vi "GCFS.vi"() -> ()   [LabVIEW 2024]
uses:
  Micro/DataCluster_GCFS.ctl
  <vilib>/userDefined/High Color/IMAQdx.ctl
  <vilib>/vision/Image Controls.llb/IMAQ Image.ctl
  <vilib>/DAQmx/read.llb/DAQmx Read (Analog DBL 1Chan 1Samp).vi
  a928a3f2-b033-44d4-bb12-0a68a29b5955.vi
  af9ea1de-6e94-45bd-9990-e3be68a33346.vi
  <vilib>/addons/_JKI Toolkits/State Machine/_JKI_lib_State_Machine.llb/Select State(s)_err__jki_lib_state_machine.vi
  acfa19c5-c678-4b0a-b648-770311154047.vi
  <extravilib>/ChannelInstances/Tag-t'DataCluster_GCFS.ctl'/Read With Abort.vi
  <extravilib>/ChannelInstances/Tag-t'DataCluster_GCFS.ctl'/Write With Abort.vi
  <extravilib>/ChannelInstances/Tag-t'DataCluster_GCFS.ctl'/Instantiate.vi
  <extravilib>/ChannelInstances/Tag-t'DataCluster_GCFS.ctl'/EndpointRead.vi
  <vilib>/DAQmx/miscellaneous.llb/DAQmx Fill In Error Info.vi
  <vilib>/addons/control/pid/pid.llb/PID (DBL).vi
  <vilib>/addons/_JKI Toolkits/State Machine/_JKI_lib_State_Machine.llb/Periodic Trigger__ogtk__JKI-SM__jki_lib_state_machine.vi
  <vilib>/Utility/file.llb/Write Delimited Spreadsheet (DBL).vi
  <vilib>/DAQmx/create/channels.llb/DAQmx Create Channel (AI-Temperature-RTD).vi
  <extravilib>/ChannelInstances/Tag-t'DataCluster_GCFS.ctl'/Endpoint.vi
  <vilib>/vision/driver/NI_Vision_Acquisition_Software.lvlib
  <extravilib>/ChannelInstances/Tag-t'DataCluster_GCFS.ctl'.lvlib
  <vilib>/addons/control/pid/NI_PID_pid.lvlib
panel:
  out "valid?":bool
  out "Waveform Chart":dbl(graph)
  in  "Load PID":bool
  in  "Tab Control":enum32{"Heating PID", "Cooling PID"}(tab)
  in  "proportional H":dbl=2.5
  in  "integral H":dbl=1.5
  in  "derivative H":dbl=0.8
  in  "proportional C":dbl=2.6
  in  "integral C":dbl=0.08
  in  "derivative C":dbl=0.1
  in  "OFF":bool
  in  "Cool":bool
  in  "Heat":bool
  in  "Cool A.":bool
  out "error out":errorcluster
  out "cDAQ Connection":bool
  out "Ready":bool
  in  "TempGrad":dbl=1.0
  in  "Get Temp":bool
  out "Temperature":dbl
  out "Data run":i32
  out "Droplet Lables":T1(plugin-control)
  in  "Grap Position Image":bool
  in  "Active":bool
  in  "Get Image":bool
  out "CAM Connection":bool
  out "UNO Connection":bool
  out "PSU Connection":bool
  out "Save loop":i32
  out "Data Loop":i32
  in  "Freezing value":sgl=250.0
  out "Frezz Image":T1(plugin-control)
  out "Droplet binary":T1(plugin-control)
  out "Grap Image":T1(plugin-control)
  in  "Sample name":string
  out "Statusstring":string
  out "Particle Measurements":dbl[][](array[numeric]) format="%.2f"
  out "Number of Particles":i32
  in  "Exit":bool
  # "Manual Controls"
  # "Temp"
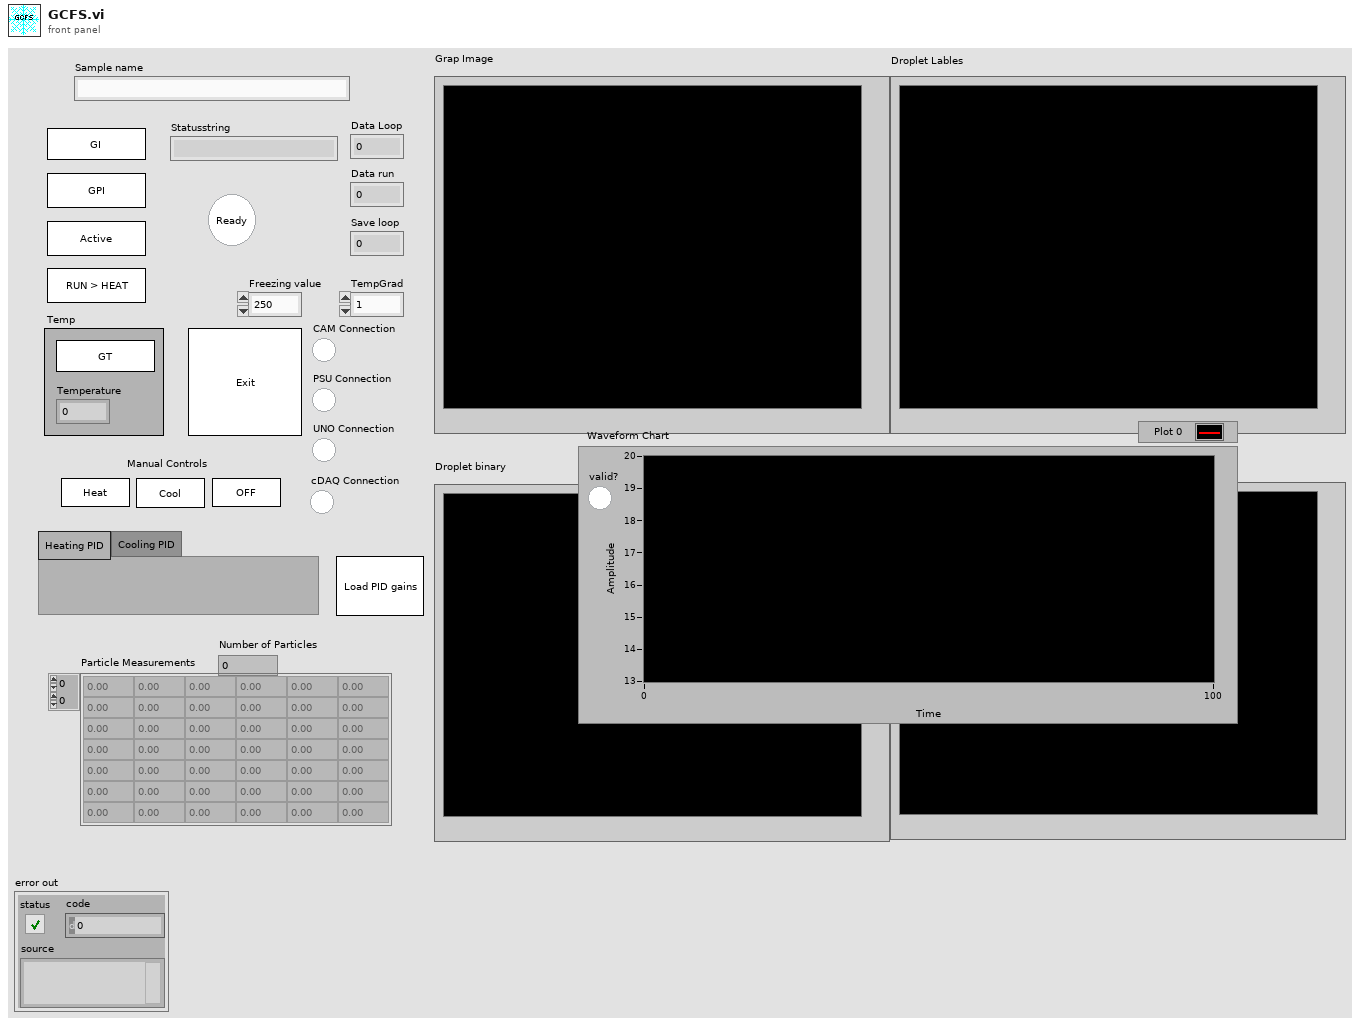
[diagram p1: front panel]
types:
  T1 = typedef "IMAQ Image.ctl" = refnum<image>
  T2 = typedef "DataCluster_GCFS.ctl" = cluster{"Core":cluster{"Current VI Reference":refnum<vi>, "Close Panel on Exit?":bool}, "Camera Cluster":cluster{"Session":T3, "Image":T1, "Position Image":T1, "PixelVal Image":T1, "Position Image Binary":T1, "Lable Image":T1, "Merged Image":T1, "Connection":bool}, "Data In Cluster":cluster{"Images":cluster{"Position Image path":path, "Sample folder path":path, "Label Image path":path}, "Sample Name":string, "Sample Rate":i32, "Gradient Buffer":i32, "Data Acquisition.Setup.TempGrad":dbl, "Control.HeatingPID gains":cluster{"proportional gain (Kc)":dbl, "integral time (Ti, min)":dbl, "derivative time (Td, min)":dbl}, "Freezing value":sgl, "Sample Rate 2":i32, "Control.CoolingPID gains":cluster{"proportional gain (Kc)":dbl, "integral time (Ti, min)":dbl, "derivative time (Td, min)":dbl}}, "Active":bool, "Ready":bool, "Exit":bool, "Arduino":cluster{"Connection":bool, "Port":refnum<visa-resource-name>, "State":string}, "Program_Start":string, "Data Out Cluster":cluster{"Particle Measurements":dbl[][], "Number of droplets":i32, "PosImg_Timestamp":string, "Que":refnum<queue>, "Lable coordinates":cluster{"X-Coordinate":i32, "Y-Coordinate":i32}[]}, "PSU":cluster{"Connection":bool, "Port":refnum<visa-resource-name>, "State":string}, "Load Rerun":bool, "Rerun":bool, "cDAQ":cluster{"Connection":bool, "ID":string, "Task":refnum<k21>}, "Temp":cluster{"Manual Temp":bool, "Target":dbl}, "Cool A.":bool}
  T3 = typedef "IMAQdx.ctl" = refnum<k21>
  T4 = enum32{"Invalid", "Standard", "Closed", "Hidden", "Minimized", "Maximized"}
  T5 = enum32{"invalid app kind", "Development System", "Run Time System", "Student Edition", "Embedded LabVIEW", "Evaluation", "Custom"}
  T6 = cluster{"Image To Save":T1, "Snap timestamp":string, "Pixel values":string[][], "Freezing points":string[][], "FreezingData":bool, "Image Pixels (U16)":u16[][]}
  T7 = cluster{"Current VI Reference":refnum<vi>, "Close Panel on Exit?":bool}
  T8 = cluster{"proportional gain (Kc)":dbl, "integral time (Ti, min)":dbl, "derivative time (Td, min)":dbl}
  T9 = typedef "Image Type" = u32
  T10 = cluster{"Type":u32, "Version":u32, "Flags":u32, "SerialNumberHigh":u32, "SerialNumberLow":u32, "BusType":u32, "InterfaceName":string, "VendorName":string, "ModelName":string, "CameraFileName":string, "CameraAttributeURL":string}[]
  T11 = typedef "Tag-t'DataCluster_GCFS.ctl'.lvlib/))Channel.ctl" = refnum<queue>
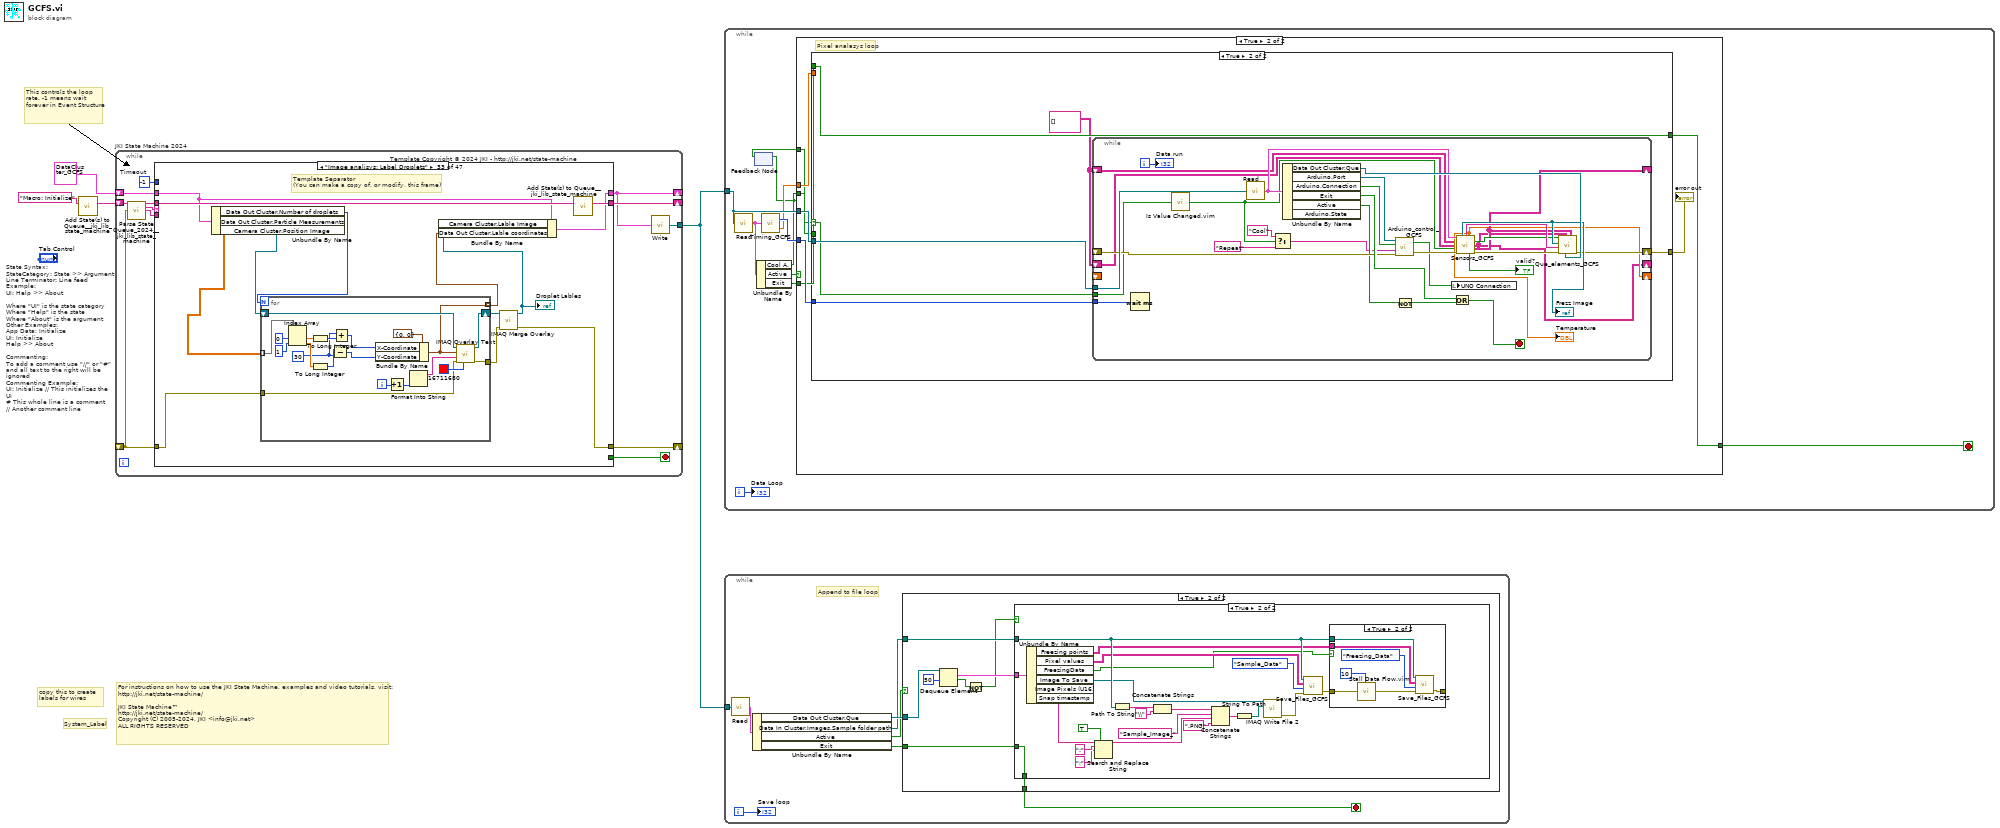
[diagram p0: block diagram]
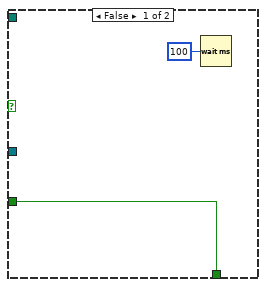
[diagram p2: hidden frame]
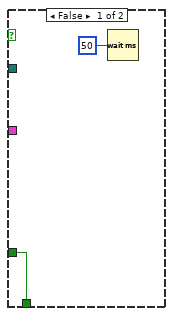
[diagram p3: hidden frame]
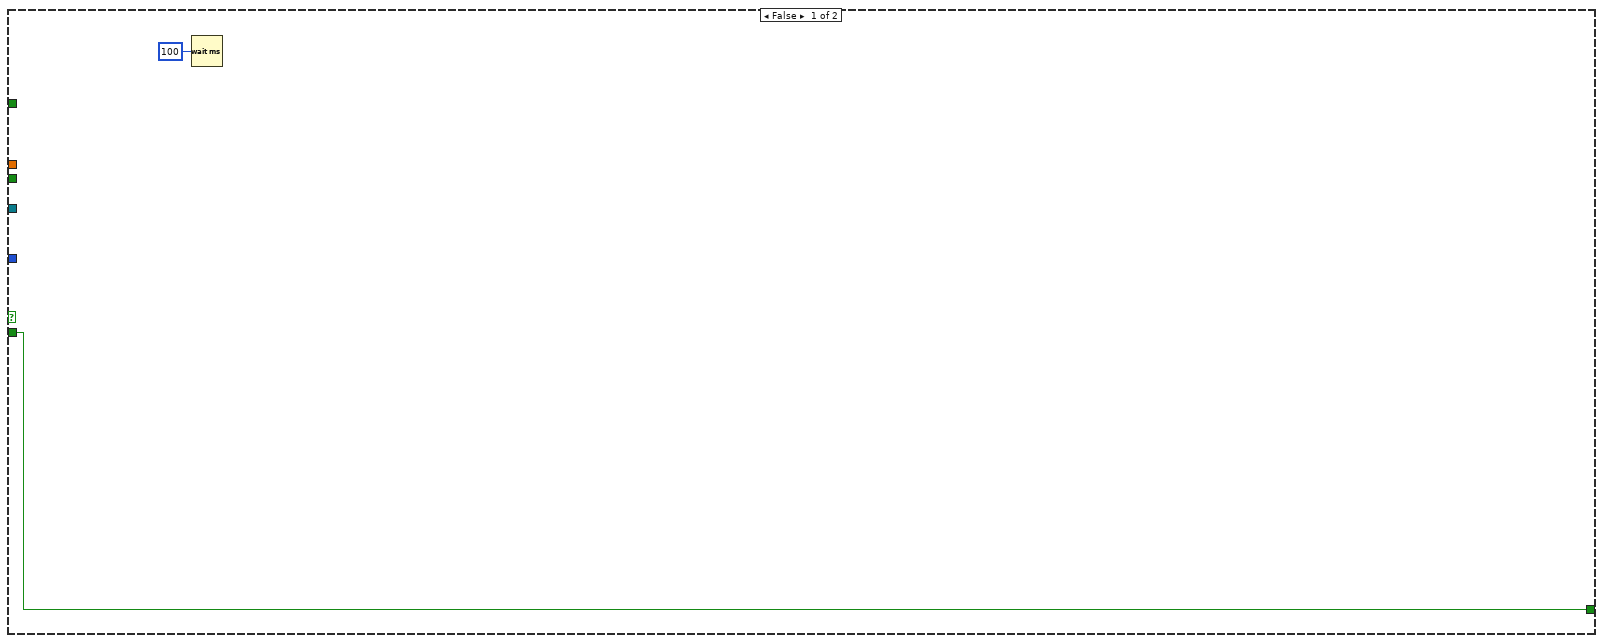
[diagram p5: hidden frame]
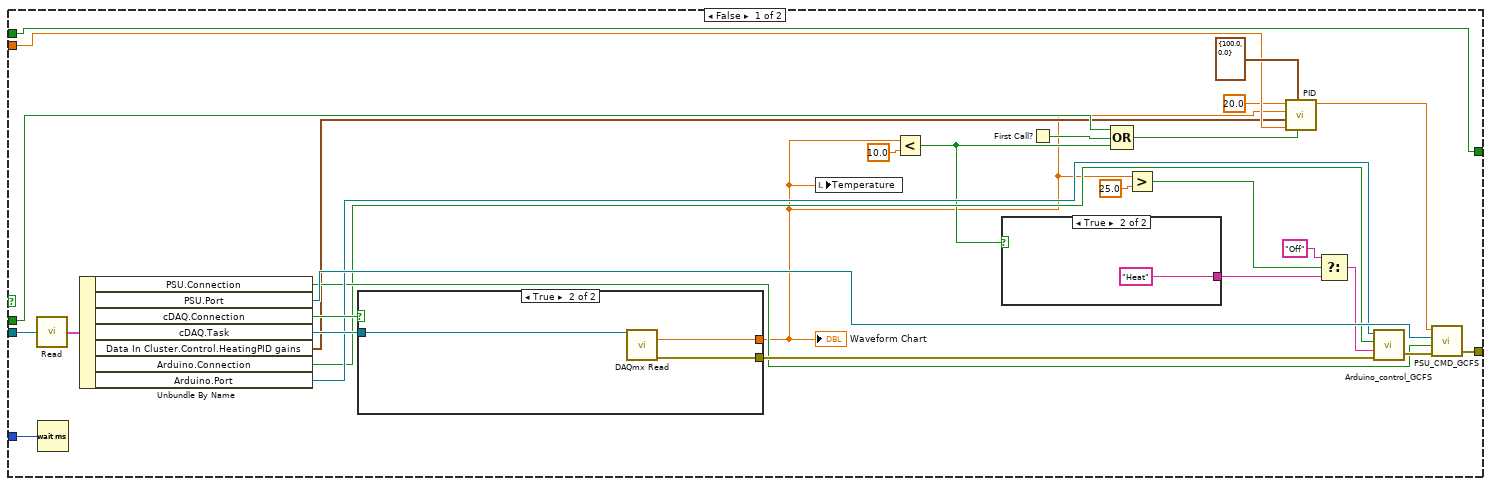
[diagram p6: hidden frame]
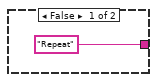
[diagram p7: hidden frame]
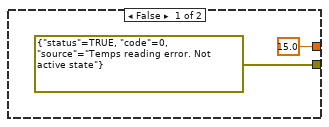
[diagram p8: hidden frame]
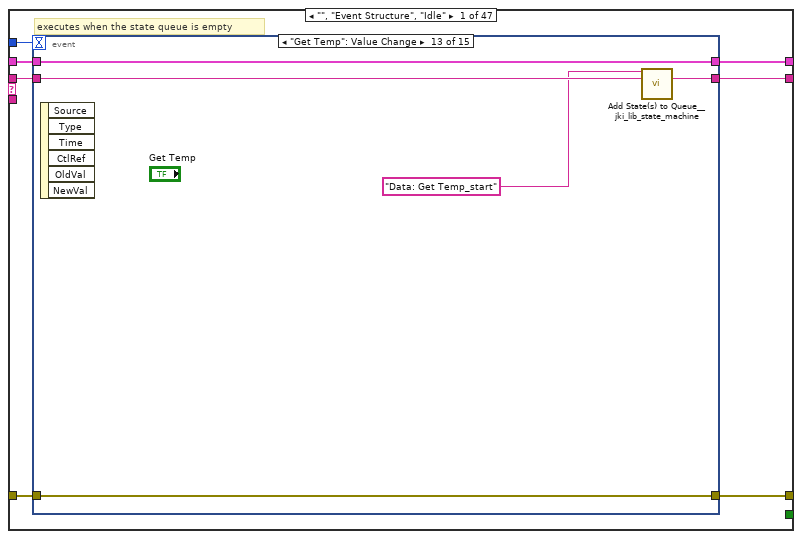
[diagram p9: hidden frame]
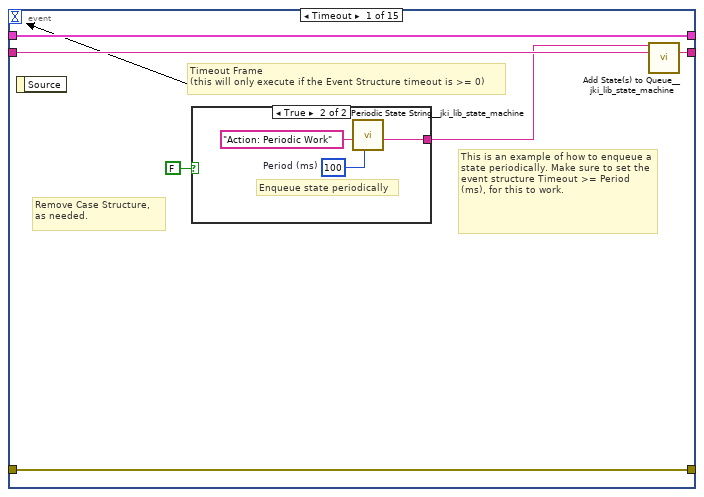
[diagram p10: hidden frame]
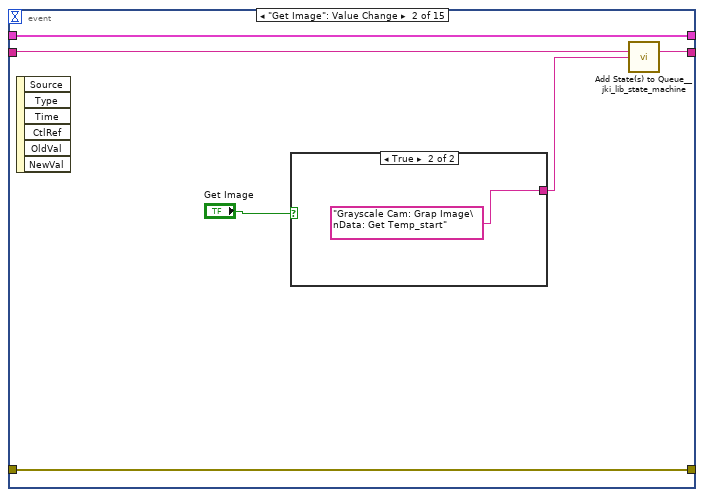
[diagram p12: hidden frame]
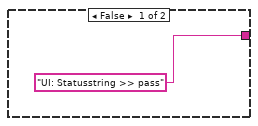
[diagram p13: hidden frame]
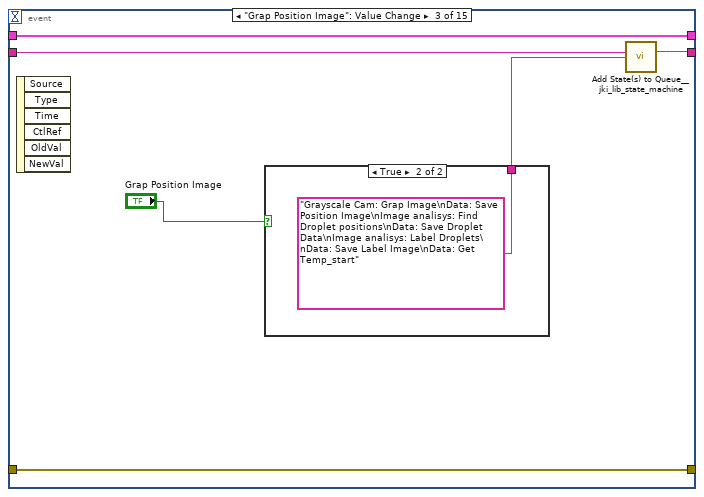
[diagram p14: hidden frame]
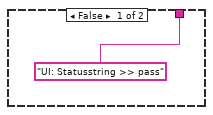
[diagram p15: hidden frame]
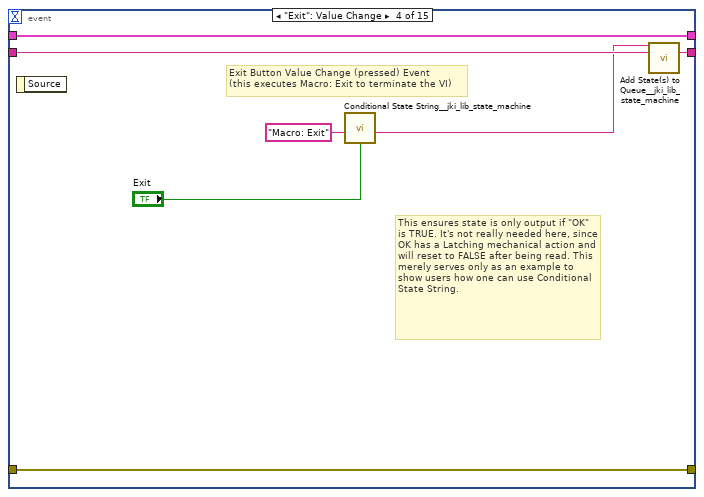
[diagram p16: hidden frame]
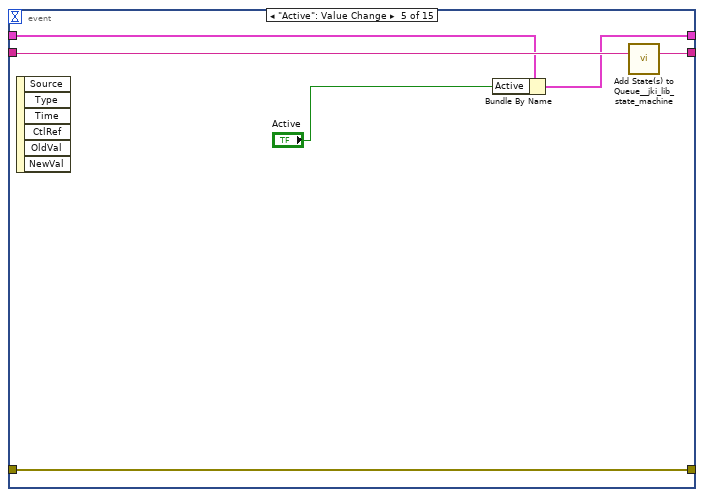
[diagram p17: hidden frame]
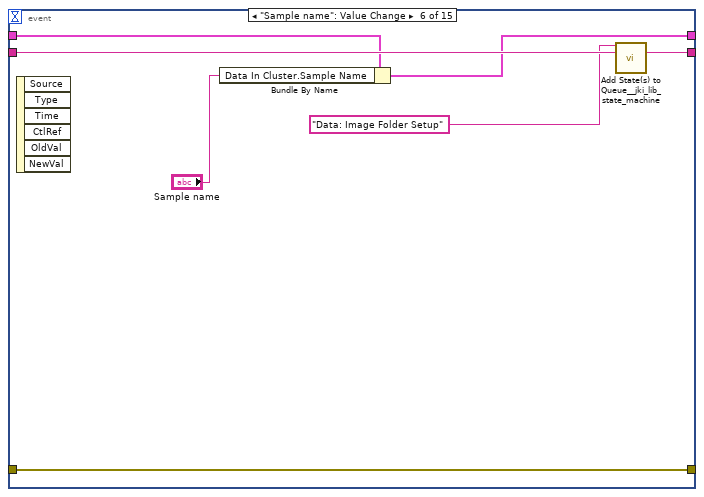
[diagram p18: hidden frame]
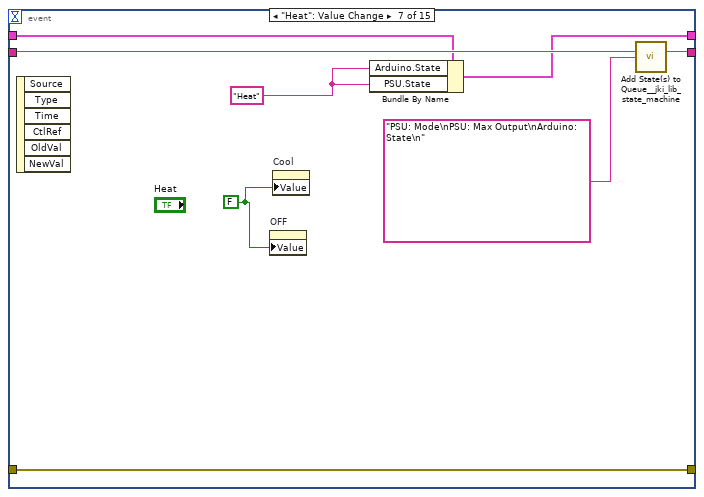
[diagram p19: hidden frame]
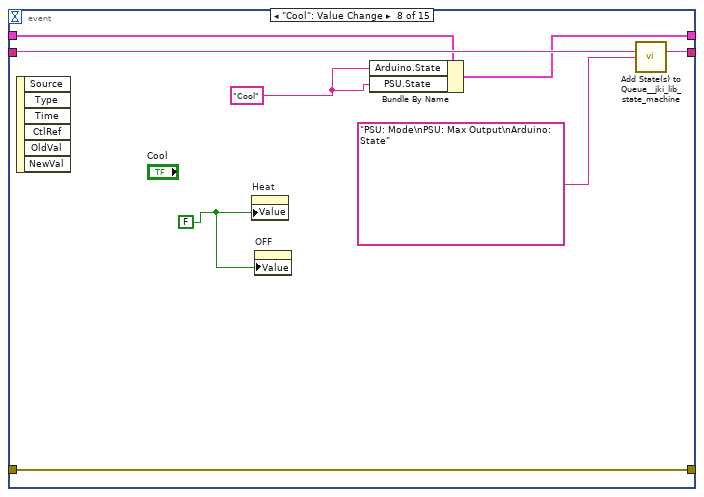
[diagram p20: hidden frame]
diagram:
  # "For instructions on how to use the JKI State Machine, examples and video tutorials, visit:\nhttp://jki.net/state-machine/\n\nJKI State Machine™\nhttp://jki.net/state-machine/\nCopyright (C) 2005-2024, JKI <info@jki.net>\nALL RIGHTS RESERVED"
  # "State Syntax:\nStateCategory: State >> Argument\nLine Terminator: Line feed\nExample:\nUI: Help >> About\n\nWhere \"UI\" is the state category\nWhere \"Help\" is the state\nWhere \"About\" is the argument\nOther Examples:\nApp Data: Initialize\nUI: Initialize\nHelp >> About\n\nCommenting:\nTo add a comment use \"//\" or \"#\" and all text to the right will be ignored\nCommenting Example:\nUI: Initialize // This initializes the UI\n# This whole line is a comment\n// Another comment line"
  # "copy this to create labels for wires"
  # "This controls the loop rate. -1 means wait forever in Event Structure"
  # "System_Label"
  n1 = call <vilib>:"Add State(s) to Queue__jki_lib_state_machine.vi"("State(s) in (\"\")"="Macro: Initialize") -> ("States Out"=w4:string)  [unwired: 14 in]
  n2 = while "JKI State Machine 2024" {
    shift-right: [w5] -> _
    shift-left: T2 {"Core"={"Current VI Reference"=refnum, "Close Panel on Exit?"=FALSE}, "Camera Cluster"={"Session"="", "Image"=refnum, "Position Image"=refnum, "PixelVal Image"=refnum, "Position Image Binary"=refnum, "Lable Image"=refnum, "Merged Image"=refnum, "Connection"=FALSE}, "Data In Cluster"={"Images"={"Position Image path"=path "", "Sample folder path"=path "", "Label Image path"=path ""}, "Sample Name"="", "Sample Rate"=20, "Gradient Buffer"=2, "Data Acquisition.Setup.TempGrad"=1.0, "Control.HeatingPID gains"={"proportional gain (Kc)"=2.5, "integral time (Ti, min)"=1.5, "derivative time (Td, min)"=0.8}, "Freezing value"=250.0, "Sample Rate 2"=20, "Control.CoolingPID gains"={"proportional gain (Kc)"=2.6, "integral time (Ti, min)"=0.08, "derivative time (Td, min)"=0.1}}, "Active"=FALSE, "Ready"=FALSE, "Exit"=FALSE, "Arduino"={"Connection"=FALSE, "Port"="", "State"=""}, "Program_Start"="", "Data Out Cluster"={"Particle Measurements"=[], "Number of droplets"=0, "PosImg_Timestamp"="", "Que"=refnum, "Lable coordinates"=[]}, "PSU"={"Connection"=FALSE, "Port"="", "State"=""}, "Load Rerun"=FALSE, "Rerun"=FALSE, "cDAQ"={"Connection"=FALSE, "ID"="", "Task"=""}, "Temp"={"Manual Temp"=FALSE, "Target"=0.0}, "Cool A."=FALSE} -> [w9]
    shift-right: [w12] -> _
    shift-left: _ -> [w7]
    shift-right: [w11] -> _
    shift-left: w4 -> [w13]
    tunnel: [w6] -> w1
    stop <- w10 stop-if-true
    w8 = -1  # Timeout
    # "Template Copyright © 2024 JKI - http://jki.net/state-machine"
    n3 = call <vilib>:"Parse State Queue_2024__jki_lib_state_machine.vi"("State Queue"=w13, "Error In (no error)"=w7) -> ("Remaining States"=w15:string, "Current State"=w16:string, "Arguments"=w14:string)  [unwired: 11 in]
    n4 = case shown="\"Image analisys: Label Droplets\"" w16 {
      selector: w16 -> [_ _ w131 _ _ _ _ _ _ _ _ _ _ _ _ _ _ _ _ _ _ _ _ _ _ _ _ _ _ _ _ _ _ _ _ _ _ _ _ _ _ _ _ _ _ _ _]
      tunnel: w15 -> [w23 w130 w135 w154 w164 w175 w179 w184 w195 w199 w213 w227 w232 w250 w270 w292 w308 w325 w329 w350 w354 w360 w371 w441 w446 w450 w465 w490 w515 w523 w535 w549 w562 w586 w594 w604 w612 w624 w632 w647 w656 w665 w674 w686 w696 w734 w742]
      tunnel: w14 -> [_ _ _ _ w159 _ _ _ _ _ _ _ _ _ _ _ _ _ _ _ _ w355 w365 w437 _ _ _ _ _ _ _ _ _ _ _ _ _ _ _ _ _ _ _ _ _ _ _]
      tunnel: w9 -> [w21 w127 w133 w147 w161 w171 w176 w181 w193 w196 w209 w224 w230 w245 w257 w282 w299 w323 w326 w348 w352 w358 w367 w438 w443 w447 w456 w481 w509 w518 w532 w545 w559 w583 w590 w600 w608 w621 w630 w643 w654 w663 w671 w683 w689 w719 w739]
      tunnel: [w20 w128 w137 w151 errorcluster {"status"=FALSE, "code"=0, "source"=""} ("error out") w173 w177 w182 w191 w197 w211 w225 w228 w246 w259 w283 w300 w309 w327 w342 w351 w356 w368 w439 w444 w448 w453 w483 w495 w520 w533 w546 w555 w584 w591 w596 w606 w622 w627 w641 w650 w659 w672 w684 w694 w716 w735] -> w12
      tunnel: w7 -> [w17 w128 w136 w151 w160 w173 w177 w182 w191 w197 w211 w225 w229 w247 w261 w284 w294 w310 w327 w344 w351 w357 w369 w439 w444 w448 w457 w485 w502 w519 w533 w537 w557 w584 w592 w597 w607 w622 w628 w642 w651 w660 w667 w684 w694 w717 w736]
      tunnel: [w22 w129 w134 w153 w163 w174 w178 w183 w194 w198 w212 w226 w231 w249 w269 w291 w307 w324 w328 w349 w353 w359 w370 w440 w445 w449 w464 w489 w514 w522 w534 w548 w561 w585 w593 w603 w611 w623 w631 w646 w655 w664 w673 w685 w695 w733 w741] -> w11
      tunnel: [_ _ _ _ _ TRUE _ _ _ _ _ _ _ _ _ _ _ _ _ _ _ _ _ _ _ _ _ _ _ _ _ _ _ _ _ _ _ _ _ _ _ _ _ _ _ _ _] -> w10
      tunnel: [w19 w127 w133 w152 w161 w170 w176 w181 w193 w196 w208 w223 w230 w245 w256 w281 w298 w323 w326 w348 w352 w358 w367 w438 w443 w447 w455 w482 w513 w521 w532 w544 w558 w583 w589 w599 w605 w621 w629 w643 w654 w663 w671 w683 w688 w718 w740] -> w5
      tunnel: w8 -> [w18 _ _ _ _ _ _ _ _ _ _ _ _ _ _ _ _ _ _ _ _ _ _ _ _ _ _ _ _ _ _ _ _ _ _ _ _ _ _ _ _ _ _ _ _ _ _]
      frame "", "Event Structure", "Idle" {
        # "executes when the state queue is empty"
        n5 = event shown="[12] \"Get Temp\": Value Change" {
          selector: _ -> [_ _ _ _ _ _ _ _ _ _ _ _ _ _ _]
          dyn-events: _ -> [_ _ _ _ _ _ _ _ _ _ _ _ _ _ _]
          timeout: w18 -> [_ _ _ _ _ _ _ _ _ _ _ _ _ _ _]
          tunnel: w23 -> [w29 w35 w44 w55 w60 w67 w75 w83 w91 w97 w100 w109 w112 w119 w125]
          tunnel: [w28 w36 w45 w54 w61 w68 w76 w84 w92 w98 w101 w108 w111 w120 w126] -> w22
          tunnel: w21 -> [w26 w37 w46 w52 w59 w65 w73 w81 w89 w95 w103 w106 w114 w116 w123]
          tunnel: [w27 w38 w41 w53 w56 w62 w74 w82 w90 w96 w102 w107 w113 w118 w121] -> w20
          tunnel: w17 -> [w27 w38 w41 w53 w56 w62 w74 w82 w90 w96 w102 w107 w113 w118 w121]
          tunnel: [w26 w37 w46 w52 w58 w64 w72 w80 w88 w94 w103 w106 w114 w117 w124] -> w19
          event Timeout {
            # "Remove Case Structure, as needed."
            # "This is an example of how to enqueue a state periodically. Make sure to set the event structure Timeout >= Period (ms), for this to work."
            # "Timeout Frame\n(this will only execute if the Event Structure timeout is >= 0)"
            n6 = event-data() -> ()  [unwired: 1 in, 1 out]
            n7 = case shown="True" FALSE {
              tunnel: [_ w32] -> w25
              frame False {
              }
              frame True {
                w30 = u32 100  # Period (ms)
                # "Enqueue state periodically"
                n8 = call <vilib>:"Periodic State String__jki_lib_state_machine.vi"("Period (ms)"=w30, "State"="Action: Periodic Work") -> ("State Out"=w32:string)  [unwired: 9 in]
              }
            }
            n9 = call <vilib>:"Add State(s) to Queue__jki_lib_state_machine.vi"("State(s) in Front (\"\")"=w25, "State(s) in (\"\")"=w29) -> ("States Out"=w28:string)  [unwired: 13 in]
          }
          event "Get Image": Value Change {
            n10 = event-data() -> ()  [unwired: 1 in, 6 out]
            n11 = case shown="True" "Get Image" {
              tunnel: ["UI: Statusstring >> pass" "Grayscale Cam: Grap Image\nData: Get Temp_start"] -> w34
              frame False {
              }
              frame True {
              }
            }
            n12 = call <vilib>:"Add State(s) to Queue__jki_lib_state_machine.vi"("State(s) in (\"\")"=w35, "State(s) at Back (\"\")"=w34) -> ("States Out"=w36:string)  [unwired: 13 in]
          }
          event "Grap Position Image": Value Change {
            n13 = event-data() -> ()  [unwired: 1 in, 6 out]
            n14 = case shown="True" "Grap Position Image" {
              tunnel: ["UI: Statusstring >> pass" "Grayscale Cam: Grap Image\nData: Save Position Image\nImage analisys: Find Droplet positions\nData: Save Droplet Data\nImage analisys: Label Droplets\nData: Save Label Image\nData: Get Temp_start"] -> w42
              frame False {
              }
              frame True {
              }
            }
            n15 = call <vilib>:"Add State(s) to Queue__jki_lib_state_machine.vi"("State(s) in (\"\")"=w44, "State(s) at Back (\"\")"=w42) -> ("States Out"=w45:string)  [unwired: 13 in]
          }
          event "Exit": Value Change {
            # "This ensures state is only output if \"OK\" is TRUE. It's not really needed here, since OK has a Latching mechanical action and will reset to FALSE after being read. This merely serves only as an example to show users how one can use Conditional State String."
            # "Exit Button Value Change (pressed) Event\n(this executes Macro: Exit to terminate the VI)"
            n16 = event-data() -> ()  [unwired: 1 in, 1 out]
            n17 = call <vilib>:"Conditional State String__jki_lib_state_machine.vi"("Do State(s)?"="Exit", "State"="Macro: Exit") -> ("State Out"=w49:string)  [unwired: 7 in]
            n18 = call <vilib>:"Add State(s) to Queue__jki_lib_state_machine.vi"("State(s) in Front (\"\")"=w49, "State(s) in (\"\")"=w55) -> ("States Out"=w54:string)  [unwired: 13 in]
          }
          event "Active": Value Change {
            n19 = event-data() -> ()  [unwired: 1 in, 6 out]
            n20 = Bundle By Name(cluster=w59, "Active"="Active") -> (w58:T2)
            n21 = call <vilib>:"Add State(s) to Queue__jki_lib_state_machine.vi"("State(s) in (\"\")"=w60) -> ("States Out"=w61:string)  [unwired: 14 in]
          }
          event "Sample name": Value Change {
            n22 = event-data() -> ()  [unwired: 1 in, 6 out]
            n23 = Bundle By Name(cluster=w65, "Data In Cluster.Sample Name"="Sample name") -> (w64:T2)
            n24 = call <vilib>:"Add State(s) to Queue__jki_lib_state_machine.vi"("State(s) in Front (\"\")"="Data: Image Folder Setup", "State(s) in (\"\")"=w67) -> ("States Out"=w68:string)  [unwired: 13 in]
          }
          event "Heat": Value Change {
            w71 = FALSE
            w69 = "Heat" ("Arduino.State")
            n25 = event-data() -> ()  [unwired: 1 in, 6 out]
            n26 = property on="OFF" class="Bool (strict)"("Value"=w71) -> ()  [unwired: 2 in, 2 out]
            n27 = property on="Cool" class="Bool (strict)"("Value"=w71) -> ()  [unwired: 2 in, 2 out]
            n28 = Bundle By Name(cluster=w73, "Arduino.State"=w69, "PSU.State"=w69) -> (w72:T2)
            n29 = call <vilib>:"Add State(s) to Queue__jki_lib_state_machine.vi"("State(s) in (\"\")"=w75, "State(s) at Back (\"\")"="PSU: Mode\nPSU: Max Output\nArduino: State\n") -> ("States Out"=w76:string)  [unwired: 13 in]
          }
          event "Cool": Value Change {
            w79 = FALSE
            w77 = "Cool" ("Arduino.State")
            n30 = event-data() -> ()  [unwired: 1 in, 6 out]
            n31 = property on="Heat" class="Bool (strict)"("Value"=w79) -> ()  [unwired: 2 in, 2 out]
            n32 = property on="OFF" class="Bool (strict)"("Value"=w79) -> ()  [unwired: 2 in, 2 out]
            n33 = Bundle By Name(cluster=w81, "Arduino.State"=w77, "PSU.State"=w77) -> (w80:T2)
            n34 = call <vilib>:"Add State(s) to Queue__jki_lib_state_machine.vi"("State(s) in (\"\")"=w83, "State(s) at Back (\"\")"="PSU: Mode\nPSU: Max Output\nArduino: State") -> ("States Out"=w84:string)  [unwired: 13 in]
          }
          event "OFF": Value Change {
            w87 = FALSE
            w85 = "OFF" ("Arduino.State")
            n35 = event-data() -> ()  [unwired: 1 in, 6 out]
            n36 = property on="Cool" class="Bool (strict)"("Value"=w87) -> ()  [unwired: 2 in, 2 out]
            n37 = property on="Heat" class="Bool (strict)"("Value"=w87) -> ()  [unwired: 2 in, 2 out]
            n38 = Bundle By Name(cluster=w89, "Arduino.State"=w85, "PSU.State"=w85) -> (w88:T2)
            n39 = call <vilib>:"Add State(s) to Queue__jki_lib_state_machine.vi"("State(s) in (\"\")"=w91, "State(s) at Back (\"\")"="PSU: Min Output\nPSU: Mode\nArduino: State") -> ("States Out"=w92:string)  [unwired: 13 in]
          }
          event "Cool A.": Value Change {
            n40 = event-data() -> ()  [unwired: 1 in, 6 out]
            n41 = Bundle By Name(cluster=w95, "Cool A."="Cool A.") -> (w94:T2)
            n42 = call <vilib>:"Add State(s) to Queue__jki_lib_state_machine.vi"("State(s) in (\"\")"=w97) -> ("States Out"=w98:string)  [unwired: 14 in]
          }
          event "Load PID": Value Change {
            n43 = event-data() -> ()  [unwired: 1 in, 6 out]
            n44 = call <vilib>:"Add State(s) to Queue__jki_lib_state_machine.vi"("State(s) in Front (\"\")"="Data: PID gains" ("State(s) in Front (\"\")"), "State(s) in (\"\")"=w100) -> ("States Out"=w101:string)  [unwired: 13 in]
          }
          event Panel Close? {
            # "Discard the event because we'll close the front panel ourselves in Macro: Exit"
            # "Close Panel button (pressed) Event\n(this executes Macro: Exit to terminate the VI)"
            n45 = event-data() -> ()  [unwired: 1 in, 1 out]
            n46 = event-data("Discard?"=TRUE) -> ()  [unwired: 1 in, 1 out]
            n47 = call <vilib>:"Add State(s) to Queue__jki_lib_state_machine.vi"("State(s) in Front (\"\")"="Macro: Exit", "State(s) in (\"\")"=w109) -> ("States Out"=w108:string)  [unwired: 13 in]
          }
          event "Get Temp": Value Change {
            n48 = event-data() -> ()  [unwired: 1 in, 6 out]
            n49 = call <vilib>:"Add State(s) to Queue__jki_lib_state_machine.vi"("State(s) in Front (\"\")"="Data: Get Temp_start" ("State(s) in Front (\"\")"), "State(s) in (\"\")"=w112) -> ("States Out"=w111:string)  [unwired: 13 in]
          }
          event "TempGrad": Value Change {
            n50 = event-data() -> ()  [unwired: 1 in, 6 out]
            n51 = Bundle By Name(cluster=w116, "Data In Cluster.Data Acquisition.Setup.TempGrad"="TempGrad") -> (w117:T2)
            n52 = call <vilib>:"Add State(s) to Queue__jki_lib_state_machine.vi"("State(s) in (\"\")"=w119) -> ("States Out"=w120:string)  [unwired: 14 in]
          }
          event "Freezing value": Value Change {
            n53 = event-data() -> ()  [unwired: 1 in, 6 out]
            n54 = Bundle By Name(cluster=w123, "Data In Cluster.Freezing value"="Freezing value") -> (w124:T2)
            n55 = call <vilib>:"Add State(s) to Queue__jki_lib_state_machine.vi"("State(s) in (\"\")"=w125) -> ("States Out"=w126:string)  [unwired: 14 in]
          }
        }
      }
      frame "---------- Core ----------" {
        # "Do not put any code in this frame.\n(it is a separator no-op)"
        n56 = call <vilib>:"Add State(s) to Queue__jki_lib_state_machine.vi"("State(s) in (\"\")"=w130) -> ("States Out"=w129:string)  [unwired: 14 in]
      }
      frame Default {
        w140 = 42 items=["No error", "Argument error", "Memory is full", "Out of zone", "End of file", "File already open", "Generic file I/O error", "File not found", "File permission error", "Disk is full", "Duplicate path", "Too many files open", "System feature not enabled", "Resource file not found", "Cannot add resource", "Resource not found", "Image not found", "Image memory error", "Pen does not exist", "Config type invalid", "Config token not found", "Config parse error", "Config memory error", "Bad external code format", "Bad external code offset", "External code not present", "Null window", "Destroy window error", "Null menu", "Print aborted", "Bad print record", "Print driver error", "Windows error during printing", "Memory error during printing", "Print dialog error", "Generic print error", "Invalid device refnum", "Device not found", "Device parameter error", "Device unit error", "Cannot open device", "Device call aborted", "Generic error", "Cancelled by user", "Object ID too low", "Object ID too high", "Object not in heap", "Unknown heap", "Unknown object (invalid DefProc)", "Unknown object (DefProc not in table)", "Message out of range", "Invalid (null) method", "Unknown message", "Manager call not supported", "Bad address", "Network operation in progress", "Network operation timed out", "Connection is busy", "Network attribute not supported", "Network error", "Address in use", "System out of memory", "Connection aborted", "Connection refused", "Not connected", "Already connected", "Connection closed", "Initialization error (interapplication manager)", "Bad occurrence", "Wait on unbound occurrence handler", "Occurrence queue overflow", "Datalog type conflict", "Unused", "Unrecognized type (interapplication manager)", "Memory corrupt", "Failed to make temporary DLL", "Old CIN version", "Drag socket not found", "Failed to load drop-object", "Failed to register OLE object", "Failed to release OLE object", "Format specifier type mismatch", "Unknown format specifier", "Too few format specifiers", "Too many format specifiers", "Scan failed", "Newer CIN version", "Error converting to variant", "Runtime menu error", "Password tampered", "Variant attribute not found", "Incompatible variant data type", "Event data is not available", "Event Store is not present", "Occurrence is not found", "Event Queue is not created", "Event info is not available", "Refnum passed is NULL", "Error retrieving Class GUID", "Error retrieving CoClass GUID", "Error retrieving TypeLib GUID.", "Bad built application magic bytes.", "Specific driver is different from the specific driver associated with the Logical Name.", "There is no session opened to the class driver.", "Max Error", "MAX - Error with config objects", "MAX - Error loading configuration", "MAX - Group not supported"]
        # "Current State"
        # "Do not delete, rename, or modify this frame.\n(this is used to capture unhandled states and typos)"
        # "Handle mistyped state name (developer tool)"
        n57 = Format Into String(format string="Software Exception: Unhandled State \"%s\"." ("message"), error in=w136, w131) -> (resulting string=w139:string, error out=w138:errorcluster)  [unwired: 1 in]
        n58 = call <vilib>:"Error Cluster From Error Code.vi"("show call chain? (False)"=TRUE, "error in (no error)"=w138, "error message (\"\")"=w139, "error code (0)"=w140) -> ("error out"=w137:errorcluster)  [unwired: 5 in]
        n59 = call <vilib>:"Add State(s) to Queue__jki_lib_state_machine.vi"("State(s) in (\"\")"=w135) -> ("States Out"=w134:string)  [unwired: 14 in]
      }
      frame "Initialize Core Data" {
        # "Do not delete, rename, or modify this frame.\n(this is used to determine panel behavior on exit)"
        # "originally closed?"
        # "exe?"
        # "If panel starts closed or is an EXE, then close it when we exit"
        n60 = property class="VI"() -> ("FP.State"=w144:T4)  [unwired: 2 in, 2 out]
        n61 = property class="App"() -> ("App.Kind"=w150:T5)  [unwired: 2 in, 2 out]
        n62 = control-ref of="Current VI Reference"() -> (w145:refnum<vi>)
        n63 = Equal?(x=w144, y=T4."Closed" ("Front Panel Window:State")) -> (x = y?=w142:bool)
        n64 = Equal?(x=w150, y=T5."Run Time System" ("Application:Kind")) -> (x = y?=w148:bool)
        n65 = Or(x=w142, y=w148) -> (x .or. y?=w146:bool)
        n66 = Bundle By Name(cluster=w147, "Core.Current VI Reference"=w145, "Core.Close Panel on Exit?"=w146) -> (w152:T2)
        n67 = call <vilib>:"Add State(s) to Queue__jki_lib_state_machine.vi"("State(s) in (\"\")"=w154) -> ("States Out"=w153:string)  [unwired: 14 in]
      }
      frame "Error Handler" {
        # "When running as sourcecode, this function will add previous state data to the error message to aid the developer in troubleshoot errors.\nIf run as an executable, no additional information is added to the error message."
        # "This state receives both Errors and Warnings which is how the Status of this wire can be FALSE"
        # "Unhandled Error -- Display it"
        # "Handle any errors or warnings here.\nYou can also output any states to clean-up after errors or warnings occur"
        # "Clear error or warning"
        n68 = disable-structure shown="Default" {
          disable-tunnel: w160 -> [w167 w168]
          disable-tunnel: w159 -> [w166 _]
          disable-tunnel: [w165 w168] -> w158
          frame condition #0 (active) {
            n69 = call <vilib>:"Append Error Details__jki_lib_state_machine.vi"("error in (no error)"=w167, "Previous State and Argument(s)"=w166) -> ("error out"=w165:errorcluster)  [unwired: 9 in]
          }
          frame condition #1 {
          }
        }
        n70 = call <vilib>:"General Error Handler.vi"("error in (no error)"=w158) -> ()  [unwired: 10 in, 5 out]
        n71 = call-poly <vilib>:"Select State(s)__jki_lib_state_machine.vi"("State(s) if True (\"\")"="/* Post Error States", "Select"=w158, "State(s) if False (\"\")"="/* Post Warning States") -> ("States Out"=w156:string)  [unwired: 12 in]
        n72 = call <vilib>:"Add State(s) to Queue__jki_lib_state_machine.vi"("State(s) in Front (\"\")"=w156, "State(s) in (\"\")"=w164) -> ("States Out"=w163:string)  [unwired: 13 in]
      }
      frame "Exit" {
        # "Do not put any code in this frame.\n(No errors that occur here will be handled.)"
        n73 = Bundle By Name(cluster=w171, "Exit"=TRUE) -> (w170:T2)
        n74 = call <vilib>:"Add State(s) to Queue__jki_lib_state_machine.vi"("State(s) in (\"\")"=w175) -> ("States Out"=w174:string)  [unwired: 14 in]
      }
      frame "---------- Macro ----------" {
        # "Do not put any code in this frame.\n(It is a separator no-op. You can make a copy of this frame to create a new Macro frame)"
        n75 = call <vilib>:"Add State(s) to Queue__jki_lib_state_machine.vi"("State(s) in (\"\")"=w179) -> ("States Out"=w178:string)  [unwired: 14 in]
      }
      frame "Macro: Initialize" {
        w180 = "UI: Initialize\nUI: Statusstring >> Initialysing\ncDAQ: Scan\ncDAQ: Initialize\nPSU: Initialize\nPSU: Mode\nArduino: Initialize\nGrayscale Cam: Initialize\nData: Initialize\nData: PID gains\nInitialize Core Data\nUI: Front Panel State >> Open\nData: Get Temp_start\nData: Image Folder Setup\nUI: Statusstring >> Initialysation done\nUI: Ready"  # UI: Initialize UI: Statusstring >> Initialysing cDAQ: Scan cDAQ: Initialize PSU: Initialize PSU: Mode Arduino: Initialize Grayscale Cam: Initialize Data: Initialize Data: PID gains Initialize Core Data UI: Front Panel State >> Open Data: Get Temp_start Data: Image Folder Setup UI: Statusstring >> Initialysation done UI: Ready
        # "Initialization Macro\n(This is called once, when the VI starts)"
        n76 = call <vilib>:"Add State(s) to Queue__jki_lib_state_machine.vi"("State(s) in Front (\"\")"=w180, "State(s) in (\"\")"=w184) -> ("States Out"=w183:string)  [unwired: 13 in]
      }
      frame "Macro: Exit" {
        w192 = "Data: Cleanup\nUI: StatusString >> Terminating cDAQ Connection (Thermistor)\ncDAQ: Terminate\nUI: StatusString >> Terminating Camera Connection\nGrayscale Cam: Terminate\nUI: StatusString >> Terminating Arduino Connection\nArduino: Terminate\nUI: StatusString >> Terminating Power Supply\nPSU: Terminate\nUI: StatusString >> See you soon\nUI: Uninitialize\nExit"  # Data: Cleanup UI: StatusString >> Terminating cDAQ Connection (Thermistor) cDAQ: Terminate UI: StatusString >> Terminating Camera Connection Grayscale Cam: Terminate UI: StatusString >> Terminating Arduino Connection Arduino: Terminate UI: StatusString >> Terminating Power Supply PSU: Terminate UI: StatusString >> See you soon UI: Uninitialize Exit
        # "Exit Macro\n(This is called once, when the VI exits)"
        n77 = Unbundle By Name(w193) -> ("Core.Close Panel on Exit?"=w189:bool)
        n78 = call <vilib>:"Conditional State String__jki_lib_state_machine.vi"("Do State(s)?"=w189, "State"="UI: Front Panel State >> Close") -> ("State Out"=w188:string)  [unwired: 7 in]
        n79 = call <vilib>:"Add State(s) to Queue__jki_lib_state_machine.vi"("State(s) in (\"\")"=w188, "State(s) at Back (\"\")"=w192) -> ("States Out"=w187:string)  [unwired: 13 in]
        n80 = call "Stall Data Flow.vim"("value in"=w187, "milliseconds to wait"=u32 50) -> ("value out"=w186:string)  [unwired: 1 out]
        n81 = call <vilib>:"Add State(s) to Queue__jki_lib_state_machine.vi"("State(s) in Front (\"\")"=w186, "State(s) in (\"\")"=w195) -> ("States Out"=w194:string)  [unwired: 13 in]
      }
      frame "---------- Data ----------" {
        # "Do not put any code in this frame.\n(It is a separator no-op. You can make a copy of this frame to create a new Data frame)"
        n82 = call <vilib>:"Add State(s) to Queue__jki_lib_state_machine.vi"("State(s) in (\"\")"=w199) -> ("States Out"=w198:string)  [unwired: 14 in]
      }
      frame "Data: Initialize" {
        w210 = T7 {"Current VI Reference"=refnum, "Close Panel on Exit?"=FALSE}  # Core
        # "do not delete - used by framework"
        # "Initialize the shift-register data, here.\n(data names are defined by what you wire into the bundle function)"
        n83 = local read "Sample name"() -> (w206:string)
        n84 = Equal?(x=w206, y="") -> (x = y?=w205:bool)
        n85 = call "Prompt User for Sample name"("Enable"=w205) -> ("Sample name"=w204:string)  [unwired: 16 in, 2 out]
        n86 = Select(t=w204, s=w205, f=w206) -> (s? t:f=w203:string)
        n87 = Obtain Queue(name (unnamed)="Save Queue", element data type=T6 {"Image To Save"=refnum, "Snap timestamp"="", "Pixel values"=[], "Freezing points"=[], "FreezingData"=FALSE, "Image Pixels (U16)"=[]}) -> (queue out=w200:refnum<queue>)  [unwired: 3 in, 2 out]
        n88 = Bundle By Name(cluster=w209, "Data Out Cluster.Que"=w200, "Core"=w210, "Data In Cluster.Sample Name"=w203) -> (w208:T2)
        n89 = local write "Sample name"(w203) -> ()
        n90 = call <vilib>:"Add State(s) to Queue__jki_lib_state_machine.vi"("State(s) in (\"\")"=w213) -> ("States Out"=w212:string)  [unwired: 14 in]
      }
      frame "Data: PID gains" {
        w222 = T8 {"proportional gain (Kc)"=0.0, "integral time (Ti, min)"=0.0, "derivative time (Td, min)"=0.0} ("Data In Cluster.Control.HeatingPID gains")
        # "Do not put any code in this frame.\n(It is a separator no-op. You can make a copy of this frame to create a new Data frame)"
        n91 = Bundle By Name(cluster=w222, "proportional gain (Kc)"="proportional H", "integral time (Ti, min)"="integral H", "derivative time (Td, min)"="derivative H") -> (w221:T8)
        n92 = Bundle By Name(cluster=w222, "proportional gain (Kc)"="proportional C", "integral time (Ti, min)"="integral C", "derivative time (Td, min)"="derivative C") -> (w220:T8)
        n93 = Bundle By Name(cluster=w224, "Data In Cluster.Control.HeatingPID gains"=w221, "Data In Cluster.Control.CoolingPID gains"=w220) -> (w223:T2)
        n94 = call <vilib>:"Add State(s) to Queue__jki_lib_state_machine.vi"("State(s) in (\"\")"=w227) -> ("States Out"=w226:string)  [unwired: 14 in]
      }
      frame "Data: Get Temp_start" {
        # "Do not put any code in this frame.\n(It is a separator no-op. You can make a copy of this frame to create a new Data frame)"
        n95 = disable-structure shown="Enabled" {
          disable-tunnel: w230 -> [_ w239]
          disable-tunnel: w229 -> [_ w236]
          disable-tunnel: [_ w235] -> w228
          frame Disabled {
            n96 = call "DAQ Assistant"("timeout (s)"=0.5) -> ("data"=w233:dynamicdata)  [unwired: 16 in, 2 out]
            n97 = local write "Temperature"(w233) -> ()
          }
          frame Enabled {
            n98 = Unbundle By Name(w239) -> ("cDAQ.Task"=w238:refnum<k21>, "cDAQ.Connection"=w237:bool)
            n99 = case shown="True" w237 {
              tunnel: w238 -> [_ w244]
              tunnel: w236 -> [w240 w243]
              tunnel: [w240 w242] -> w235
              frame False {
              }
              frame True {
                n100 = call-poly <vilib>:"DAQmx Read.vi"("task/channels in"=w244, "error in"=w243) -> ("data"=w241:dbl, "error out"=w242:errorcluster)  [unwired: 11 in, 1 out]
                n101 = local write "Temperature"(w241) -> ()
              }
            }
          }
        }
        n102 = call <vilib>:"Add State(s) to Queue__jki_lib_state_machine.vi"("State(s) in (\"\")"=w232) -> ("States Out"=w231:string)  [unwired: 14 in]
      }
      frame "Data: Cleanup" {
        # "Cleanup any data and references, here.\n(this is called automatically, by the Macro: Exit)"
        n103 = Unbundle By Name(w245) -> ("Core.Current VI Reference"=w248:refnum<vi>)
        n104 = Close Reference(reference=w248, error in (no error)=w247) -> (error out=w246:errorcluster)
        n105 = call <vilib>:"Add State(s) to Queue__jki_lib_state_machine.vi"("State(s) in (\"\")"=w250) -> ("States Out"=w249:string)  [unwired: 14 in]
      }
      frame "Data: Image Folder Setup" {
        w252 = "\\" ("string")
        # "Do not put any code in this frame.\n(It is a separator no-op. You can make a copy of this frame to create a new Data frame)"
        n106 = Unbundle By Name(w257) -> ("Data In Cluster.Sample Name"=w258:string)
        n107 = Format Date/Time String(time format string (%c)="%Y-%m-%d_%H;%M", UTC format=FALSE) -> (date/time string=w251:string)  [unwired: 1 in]
        n108 = call <vilib>:"Application Directory.vi"() -> ("Application Directory"=w267:path)
        n109 = Path To String(path=w267) -> (string=w266:string)
        n110 = Concatenate Strings(w266, w252, "Flat Surface Images" ("string"), w252, w258, w252, w251) -> (w264:string)
        n111 = String To Path(string=w264) -> (path=w265:path)
        n112 = call <vilib>:"Check if File or Folder Exists.vi"("error in (no error)"=w261, "path"=w265) -> ("error out"=w260:errorcluster, "file or folder exists?"=w263:bool, "dup path"=w262:path)  [unwired: 7 in]
        n113 = case shown="False" w263 {
          tunnel: w262 -> [w272 w276]
          tunnel: w260 -> [w274 w275]
          tunnel: [w273 w275] -> w259
          tunnel: [w271 w276] -> w255
          frame False {
            n114 = Create Folder(path (use dialog)=w272, error in=w274) -> (created path=w271:path, error out=w273:errorcluster)  [unwired: 1 in, 1 out]
          }
          frame True {
          }
        }
        n115 = Bundle By Name(cluster=w257, "Data In Cluster.Images.Sample folder path"=w255, "Program_Start"=w251) -> (w256:T2)
        n116 = call <vilib>:"Add State(s) to Queue__jki_lib_state_machine.vi"("State(s) in (\"\")"=w270) -> ("States Out"=w269:string)  [unwired: 14 in]
      }
      frame "Data: Save Position Image" {
        # "Do not put any code in this frame.\n(It is a separator no-op. You can make a copy of this frame to create a new Data frame)"
        n117 = Unbundle By Name(w282) -> ("Camera Cluster.Image"=w278:T1, "Data In Cluster.Images.Sample folder path"=w286:path, "Data Out Cluster.PosImg_Timestamp"=w285:string)
        n118 = Path To String(path=w286) -> (string=w287:string)
        n119 = Concatenate Strings(w287, "\\" ("string"), "Position_Image_" ("string"), w285, ".PNG" ("string")) -> (w290:string)
        n120 = String To Path(string=w290) -> (path=w280:path)
        n121 = call-poly "IMAQ Write File 2"("error in (no error)"=w284, "File Path"=w280, "Image"=w278) -> ("error out"=w283:errorcluster, "Image Out (duplicate)"=w277:T1)  [unwired: 7 in]
        n122 = Bundle By Name(cluster=w282, "Data In Cluster.Images.Position Image path"=w280, "Camera Cluster.Position Image"=w277) -> (w281:T2)
        n123 = local write "Droplet Lables"(w277) -> ()
        n124 = call <vilib>:"Add State(s) to Queue__jki_lib_state_machine.vi"("State(s) in (\"\")"=w292) -> ("States Out"=w291:string)  [unwired: 14 in]
      }
      frame "Data: Save Label Image" {
        # "Do not put any code in this frame.\n(It is a separator no-op. You can make a copy of this frame to create a new Data frame)"
        n125 = Unbundle By Name(w299) -> ("Camera Cluster.Lable Image"=w295:T1, "Data In Cluster.Images.Sample folder path"=w302:path, "Data Out Cluster.PosImg_Timestamp"=w301:string)
        n126 = Path To String(path=w302) -> (string=w303:string)
        n127 = Concatenate Strings(w303, "\\" ("string"), "Label_Image_" ("string"), w301, ".PNG" ("string")) -> (w306:string)
        n128 = String To Path(string=w306) -> (path=w297:path)
        n129 = call-poly "IMAQ Write File 2"("error in (no error)"=w294, "File Path"=w297, "Image"=w295) -> ("error out"=w300:errorcluster, "Image Out (duplicate)"=w293:T1)  [unwired: 7 in]
        n130 = Bundle By Name(cluster=w299, "Data In Cluster.Images.Label Image path"=w297, "Camera Cluster.Merged Image"=w293) -> (w298:T2)
        n131 = call <vilib>:"Add State(s) to Queue__jki_lib_state_machine.vi"("State(s) in (\"\")"=w308) -> ("States Out"=w307:string)  [unwired: 14 in]
      }
      frame "Data: Save Droplet Data" {
        # "Do not put any code in this frame.\n(It is a separator no-op. You can make a copy of this frame to create a new Data frame)"
        n132 = Unbundle By Name(w323) -> ("Data Out Cluster.Particle Measurements"=w311:dbl[][], "Data In Cluster.Images.Sample folder path"=w322:path)
        n133 = Path To String(path=w322) -> (string=w316:string)
        n134 = Concatenate Strings(w316, "\\" ("string"), "Droplet_data" ("string"), ".csv" ("string")) -> (w321:string)
        n135 = String To Path(string=w321) -> (path=w314:path)
        n136 = call "DropletFile_Headers_GCFS.vi"("error in (no error)"=w310, "path"=w314) -> ("error out"=w312:errorcluster, "File path"=w313:path)
        n137 = call-poly <vilib>:"Write Delimited Spreadsheet.vi"("file path (dialog if empty)"=w313, "2D data"=w311, "append to file? (new file:F)"=TRUE, "error in (no error)"=w312, "delimiter (\\t)"=";" ("delimiter (\\t)")) -> ("error out"=w309:errorcluster)  [unwired: 9 in, 1 out]
        n138 = call <vilib>:"Add State(s) to Queue__jki_lib_state_machine.vi"("State(s) in (\"\")"=w325) -> ("States Out"=w324:string)  [unwired: 14 in]
      }
      frame "---------- UI ----------" {
        # "Do not put any code in this frame.\n(It is a separator no-op. You can make a copy of this frame to create a new UI frame)"
        n139 = call <vilib>:"Add State(s) to Queue__jki_lib_state_machine.vi"("State(s) in (\"\")"=w329) -> ("States Out"=w328:string)  [unwired: 14 in]
      }
      frame "UI: Initialize" {
        w330 = FALSE
        w332 = 0 ("Number of Particles")
        w331 = FALSE ("Cool")
        w338 = "\\" ("string")
        w346 = T9 6 items=["Grayscale (U8)", "Grayscale (I16)", "Grayscale (SGL)", "Complex (CSG)", "RGB (U32)", "HSL (U32)", "RGB (U64)", "Grayscale (U16)"] ("Image Type")
        w333 = T1 refnum ("Image")
        # "Initialize the User Interface, here.\n(this is called automatically, by the Macro: Initialize)"
        n140 = call <vilib>:"Application Directory.vi"() -> ("Application Directory"=w341:path)
        n141 = Path To String(path=w341) -> (string=w340:string)
        n142 = Concatenate Strings(w340, w338, "resources" ("string"), w338, "Logo_Full.png" ("string")) -> (w336:string)
        n143 = String To Path(string=w336) -> (path=w335:path)
        n144 = local write "Number of Particles"(w332) -> ()
        n145 = local write "Data run"(w332) -> ()
        n146 = call "IMAQ Create"("Image Name"="Logo", "Image Type"=w346, "error in (no error)"=w344) -> ("New Image"=w345:T1, "error out"=w343:errorcluster)  [unwired: 2 in]
        n147 = property on="Cool" class="Bool (strict)"("Value"=w331) -> ()  [unwired: 2 in, 2 out]
        n148 = property on="OFF" class="Bool (strict)"("Value"=w331) -> ()  [unwired: 2 in, 2 out]
        n149 = call "IMAQ ReadFile 2"("File Path"=w335, "error in (no error)"=w343, "Image"=w345) -> ("error out"=w342:errorcluster)  [unwired: 4 in, 4 out]
        n150 = property on="Heat" class="Bool (strict)"("Value"=w331) -> ()  [unwired: 2 in, 2 out]
        n151 = property on="Active" class="Bool (strict)"("Value"=w331) -> ()  [unwired: 2 in, 2 out]
        n152 = property on="Particle Measurements" class="Arr (strict)"("Value"=dbl[][] [] ("Particle Measurements (Pixels) (Particle Analysis 1)")) -> ()  [unwired: 2 in, 2 out]
        n153 = local write "Droplet binary"(w333) -> ()
        n154 = local write "Grap Image"(w333) -> ()
        n155 = local write "Frezz Image"(w333) -> ()
        n156 = local write "Ready"(w330) -> ()
        n157 = local write "PSU Connection"(w330) -> ()
        n158 = local write "UNO Connection"(w330) -> ()
        n159 = local write "CAM Connection"(w330) -> ()
        n160 = local write "cDAQ Connection"(w330) -> ()
        n161 = local write "Droplet Lables"(w333) -> ()
        n162 = call <vilib>:"Add State(s) to Queue__jki_lib_state_machine.vi"("State(s) in (\"\")"=w350) -> ("States Out"=w349:string)  [unwired: 14 in]
      }
      frame "UI: Uninitialize" {
        # "Cleanup the User Interface, here.\n(this is called automatically, by the Macro: Exit)"
        n163 = call <vilib>:"Add State(s) to Queue__jki_lib_state_machine.vi"("State(s) in (\"\")"=w354) -> ("States Out"=w353:string)  [unwired: 14 in]
      }
      frame "UI: Cursor Set" {
        # "Argument"
        # "Set and Unset Cursor Busy.\n(Usage: \"UI: Cursor Set >> Busy|Idle\")"
        n164 = case shown="\"Idle\", Default" w355 {
          tunnel: w357 -> [w362 w364]
          tunnel: [w361 w363] -> w356
          frame "Idle", Default {
            n165 = call <vilib>:"Unset Busy.vi"("error in (no error)"=w362) -> ("error out"=w361:errorcluster)  [unwired: 10 in]
          }
          frame "Busy" {
            n166 = call <vilib>:"Set Busy.vi"("error in (no error)"=w364) -> ("error out"=w363:errorcluster)  [unwired: 9 in, 1 out]
          }
        }
        n167 = call <vilib>:"Add State(s) to Queue__jki_lib_state_machine.vi"("State(s) in (\"\")"=w360) -> ("States Out"=w359:string)  [unwired: 14 in]
      }
      frame "UI: Front Panel State" {
        # "Argument"
        # "Set Front Panel Open or Closed\n(Usage: \"UI: Front Panel State >> Open|Close\")"
        n168 = Unbundle By Name(w367) -> ("Core.Current VI Reference"=w366:refnum<vi>)
        n169 = case shown="\"Open\", \"Standard\", Default" w365 {
          tunnel: w369 -> [w377 w392 w403 w416 w429]
          tunnel: [w379 w393 w405 w418 w431] -> w368
          tunnel: w366 -> [w378 w390 w404 w417 w430]
          frame "Open", "Standard", Default {
            w372 = T4."Standard" ("State")
            n170 = property class="VI"(reference=w378, error in=w377) -> (reference out=w375:refnum<vi>, error out=w376:errorcluster, "FP.State"=w374:T4)
            n171 = Not Equal?(x=w374, y=w372) -> (x != y?=w373:bool)
            n172 = case shown="True" w373 {
              tunnel: [w383 w385] -> w379
              tunnel: w376 -> [w382 w385]
              tunnel: w375 -> [w381 _]
              tunnel: w372 -> [w380 _]
              frame True {
                n173 = invoke class="VI" method="FP.Open"(reference=w381, error in=w382, "Activate"=TRUE, "State"=w380) -> (error out=w383:errorcluster)  [unwired: 1 in, 4 out]
              }
              frame False {
              }
            }
          }
          frame "Close", "Closed" {
            n174 = property class="VI"(reference=w390, error in=w392) -> (reference out=w389:refnum<vi>, error out=w391:errorcluster, "FP.State"=w387:T4)
            n175 = Not Equal?(x=w387, y=T4."Closed" ("Front Panel Window:State")) -> (x != y?=w386:bool)
            n176 = case shown="True" w386 {
              tunnel: [w394 w397] -> w393
              tunnel: w391 -> [w394 w396]
              tunnel: w389 -> [_ w395]
              frame False {
              }
              frame True {
                n177 = invoke class="VI" method="FP.Close"(reference=w395, error in=w396) -> (error out=w397:errorcluster)  [unwired: 1 in, 2 out]
              }
            }
          }
          frame "Hidden", "Hide" {
            w398 = T4."Hidden" ("State")
            n178 = property class="VI"(reference=w404, error in=w403) -> (reference out=w401:refnum<vi>, error out=w402:errorcluster, "FP.State"=w400:T4)
            n179 = Not Equal?(x=w400, y=w398) -> (x != y?=w399:bool)
            n180 = case shown="True" w399 {
              tunnel: [w409 w410] -> w405
              tunnel: w402 -> [w408 w410]
              tunnel: w401 -> [w407 _]
              tunnel: w398 -> [w406 _]
              frame True {
                n181 = invoke class="VI" method="FP.Open"(reference=w407, error in=w408, "State"=w406) -> (error out=w409:errorcluster)  [unwired: 2 in, 4 out]
              }
              frame False {
              }
            }
          }
          frame "Minimize", "Minimized" {
            w411 = T4."Minimized" ("State")
            n182 = property class="VI"(reference=w417, error in=w416) -> (reference out=w414:refnum<vi>, error out=w415:errorcluster, "FP.State"=w413:T4)
            n183 = Not Equal?(x=w413, y=w411) -> (x != y?=w412:bool)
            n184 = case shown="True" w412 {
              tunnel: [w422 w423] -> w418
              tunnel: w415 -> [w421 w423]
              tunnel: w414 -> [w420 _]
              tunnel: w411 -> [w419 _]
              frame True {
                n185 = invoke class="VI" method="FP.Open"(reference=w420, error in=w421, "State"=w419) -> (error out=w422:errorcluster)  [unwired: 2 in, 4 out]
              }
              frame False {
              }
            }
          }
          frame "Maximize", "Maximized" {
            w424 = T4."Maximized" ("State")
            n186 = property class="VI"(reference=w430, error in=w429) -> (reference out=w427:refnum<vi>, error out=w428:errorcluster, "FP.State"=w426:T4)
            n187 = Not Equal?(x=w426, y=w424) -> (x != y?=w425:bool)
            n188 = case shown="True" w425 {
              tunnel: [w435 w436] -> w431
              tunnel: w428 -> [w434 w436]
              tunnel: w427 -> [w433 _]
              tunnel: w424 -> [w432 _]
              frame True {
                n189 = invoke class="VI" method="FP.Open"(reference=w433, error in=w434, "State"=w432) -> (error out=w435:errorcluster)  [unwired: 2 in, 4 out]
              }
              frame False {
              }
            }
          }
        }
        n190 = call <vilib>:"Add State(s) to Queue__jki_lib_state_machine.vi"("State(s) in (\"\")"=w371) -> ("States Out"=w370:string)  [unwired: 14 in]
      }
      frame "UI: Statusstring" {
        # "Do not put any code in this frame.\n(It is a separator no-op. You can make a copy of this frame to create a new UI frame)"
        n191 = call <vilib>:"Add State(s) to Queue__jki_lib_state_machine.vi"("State(s) in (\"\")"=w441) -> ("States Out"=w440:string)  [unwired: 14 in]
        "Statusstring" <- w437
      }
      frame "UI: Ready" {
        # "Do not put any code in this frame.\n(It is a separator no-op. You can make a copy of this frame to create a new UI frame)"
        n192 = call <vilib>:"Add State(s) to Queue__jki_lib_state_machine.vi"("State(s) in (\"\")"=w446) -> ("States Out"=w445:string)  [unwired: 14 in]
        "Ready" <- TRUE ("Ready")
      }
      frame "---------- Grayscale Cam ----------" {
        # "Template Separator\n(You can make a copy of, or modify, this frame)"
        n193 = call <vilib>:"Add State(s) to Queue__jki_lib_state_machine.vi"("State(s) in (\"\")"=w450) -> ("States Out"=w449:string)  [unwired: 14 in]
      }
      frame "Grayscale Cam: Initialize" {
        # "Template Separator\n(You can make a copy of, or modify, this frame)"
        n194 = call <vilib>:"IMAQdx Enumerate Cameras.vi"("error in"=w457) -> ("error out"=w458:errorcluster, "Camera Information Array"=w462:T10)  [unwired: 9 in]
        n195 = Array Size(array=w462) -> (size(s)=w463:i32)
        n196 = for {
          N: w463 -> [_]
          tunnel: w462 -> [w473] mode=indexing
          shift-right: [w471] -> w461
          shift-left: _ -> [w466]
          n197 = Unbundle By Name(w473) -> ("InterfaceName"=w472:string, "VendorName"=w470:string)
          n198 = Match True/False String(2:"" ("false string"), 3:"JAI" ("true string"), 4:w470) -> (0:w467:bool)  [unwired: 1 out]
          n199 = Select(t=w472, s=w467, f=w466) -> (s? t:f=w471:string)
        }
        n200 = call <vilib>:"IMAQdx Open Camera.vi"("error in"=w458, "Session In"=w461) -> ("error out"=w460:errorcluster, "Session Out"=w459:T3)  [unwired: 8 in]
        n201 = call <vilib>:"IMAQdx Configure Grab.vi"("error in"=w460, "Session In"=w459) -> ("error out"=w453:errorcluster, "Session Out"=w454:T3)  [unwired: 8 in]
        n202 = Unbundle By Name(w453) -> ("status"=w452:bool)
        n203 = Not(x=w452) -> (.not. x?=w451:bool)
        "CAM Connection" <- w451
        n204 = Bundle By Name(cluster=w456, "Camera Cluster.Session"=w454, "Camera Cluster.Connection"=w451) -> (w455:T2)
        n205 = call <vilib>:"Add State(s) to Queue__jki_lib_state_machine.vi"("State(s) in (\"\")"=w465) -> ("States Out"=w464:string)  [unwired: 14 in]
      }
      frame "Grayscale Cam: Grap Image" {
        w487 = T9 0 items=["Grayscale (U8)", "Grayscale (I16)", "Grayscale (SGL)", "Complex (CSG)", "RGB (U32)", "HSL (U32)", "RGB (U64)", "Grayscale (U16)"] ("Image Type")
        # "Template Separator\n(You can make a copy of, or modify, this frame)"
        n206 = Unbundle By Name(w481) -> ("Camera Cluster.Session"=w480:T3)
        n207 = call "IMAQ Create"("Image Name"="Image", "Image Type"=w487, "error in (no error)"=w485) -> ("New Image"=w486:T1, "error out"=w484:errorcluster)  [unwired: 2 in]
        n208 = Format Date/Time String(time format string (%c)="%Y-%m-%d_%H;%M;%S%3u", UTC format=FALSE) -> (date/time string=w475:string)  [unwired: 1 in]
        n209 = call <vilib>:"IMAQdx Grab2.vi"("Timeout (ms)"=5000, "error in"=w484, "Image In"=w486, "Session In"=w480) -> ("error out"=w483:errorcluster, "Image Out"=w474:T1, "Session Out"=w479:T3)  [unwired: 4 in, 1 out]
        "Grap Image" <- w474
        n210 = Bundle By Name(cluster=w481, "Camera Cluster.Session"=w479, "Camera Cluster.Image"=w474, "Data Out Cluster.PosImg_Timestamp"=w475) -> (w482:T2)
        n211 = call <vilib>:"Add State(s) to Queue__jki_lib_state_machine.vi"("State(s) in (\"\")"=w490) -> ("States Out"=w489:string)  [unwired: 14 in]
      }
      frame "Grayscale Cam: Select Test Image" {
        w499 = T9 1 items=["Grayscale (U8)", "Grayscale (I16)", "Grayscale (SGL)", "Complex (CSG)", "RGB (U32)", "HSL (U32)", "RGB (U64)", "Grayscale (U16)"] ("Image Type")
        w504 = "\\" ("string")
        # "Template Separator\n(You can make a copy of, or modify, this frame)"
        n212 = call <vilib>:"Application Directory.vi"() -> ("Application Directory"=w507:path)
        n213 = Path To String(path=w507) -> (string=w506:string)
        n214 = Concatenate Strings(w506, w504, "Flat Surface Images" ("string"), w504) -> (w505:string)
        n215 = String To Path(string=w505) -> (path=w503:path)
        n216 = call "File Dialog"("start path"=w503, "error in"=w502, "pattern (all files)"="*.png*") -> ("selected path"=w501:path, "error out"=w497:errorcluster)  [unwired: 9 in, 2 out]
        n217 = call "IMAQ Create"("Image Name"="Test", "Image Type"=w499, "error in (no error)"=w497) -> ("New Image"=w498:T1, "error out"=w496:errorcluster)  [unwired: 2 in]
        n218 = Format Date/Time String(time format string (%c)="%Y-%m-%d_%H;%M;%S%3u", UTC format=FALSE) -> (date/time string=w493:string)  [unwired: 1 in]
        n219 = call "IMAQ ReadFile 2"("File Path"=w501, "error in (no error)"=w496, "Image"=w498) -> ("error out"=w495:errorcluster, "Image Out"=w494:T1)  [unwired: 4 in, 3 out]
        n220 = Concatenate Strings("TEST_" ("string"), w493) -> (w491:string)
        n221 = Bundle By Name(cluster=w509, "Camera Cluster.Image"=w494, "Data Out Cluster.PosImg_Timestamp"=w491) -> (w513:T2)
        n222 = local write "Grap Image"(w494) -> ()
        n223 = call <vilib>:"Add State(s) to Queue__jki_lib_state_machine.vi"("State(s) in (\"\")"=w515) -> ("States Out"=w514:string)  [unwired: 14 in]
      }
      frame "Grayscale Cam: Terminate" {
        # "Template Separator\n(You can make a copy of, or modify, this frame)"
        n224 = Unbundle By Name(w518) -> ("Camera Cluster.Session"=w517:T3, "Camera Cluster.Connection"=w516:bool)
        n225 = case shown="True" w516 {
          tunnel: w517 -> [_ w529]
          tunnel: w518 -> [w525 w531]
          tunnel: [w525 w530] -> w521
          tunnel: [w524 w528] -> w520
          tunnel: w519 -> [w524 w527]
          frame False {
          }
          frame True {
            w526 = FALSE ("Connections.cDAQ.Connected")
            n226 = call <vilib>:"IMAQdx Close Camera.vi"("error in"=w527, "Session In"=w529) -> ("error out"=w528:errorcluster)  [unwired: 9 in]
            n227 = local write "CAM Connection"(w526) -> ()
            n228 = Bundle By Name(cluster=w531, "Camera Cluster.Connection"=w526) -> (w530:T2)
          }
        }
        n229 = call <vilib>:"Add State(s) to Queue__jki_lib_state_machine.vi"("State(s) in (\"\")"=w523) -> ("States Out"=w522:string)  [unwired: 14 in]
      }
      frame "---------- Image analisys ----------" {
        # "Template Separator\n(You can make a copy of, or modify, this frame)"
        n230 = call <vilib>:"Add State(s) to Queue__jki_lib_state_machine.vi"("State(s) in (\"\")"=w535) -> ("States Out"=w534:string)  [unwired: 14 in]
      }
      frame "Image analisys: Find Droplet positions" {
        w538 = T9 0 items=["Grayscale (U8)", "Grayscale (I16)", "Grayscale (SGL)", "Complex (CSG)", "RGB (U32)", "HSL (U32)", "RGB (U64)", "Grayscale (U16)"] ("Image Type")
        # "Your code here.\n(You can make a copy of, or modify, this frame)"
        n231 = Unbundle By Name(w545) -> ("Camera Cluster.Position Image"=w547:T1)
        n232 = call "IMAQ Create"("Image Name"="Binary", "Image Type"=w538, "error in (no error)"=w537) -> ("New Image"=w539:T1, "error out"=w536:errorcluster)  [unwired: 2 in]
        n233 = call "Vision Assistant"("Image In"=w547, "Image Dst"=w539, "error in"=w536) -> ("Image Out"=w541:T1, "Number of Particles (Particle Analysis 1)"=w543:i32, "Particle Measurements (Pixels) (Particle Analysis 1)"=w542:dbl[][], "error out"=w546:errorcluster)  [unwired: 19 in, 2 out]
        "Number of Particles" <- w543
        "Particle Measurements" <- w542
        "Droplet binary" <- w541
        n234 = Bundle By Name(cluster=w545, "Camera Cluster.Position Image Binary"=w541, "Data Out Cluster.Particle Measurements"=w542, "Data Out Cluster.Number of droplets"=w543) -> (w544:T2)
        n235 = call <vilib>:"Add State(s) to Queue__jki_lib_state_machine.vi"("State(s) in (\"\")"=w549) -> ("States Out"=w548:string)  [unwired: 14 in]
      }
      frame "Image analisys: Label Droplets" {
        # "Template Separator\n(You can make a copy of, or modify, this frame)"
        n236 = Unbundle By Name(w559) -> ("Data Out Cluster.Number of droplets"=w551:i32, "Data Out Cluster.Particle Measurements"=w560:dbl[][], "Camera Cluster.Position Image"=w556:T1)
        n237 = for {
          N: w551 -> [_]
          tunnel: w557 -> [w574]
          shift-right: [w569] -> w553
          shift-left: w556 -> [w570]
          tunnel: w560 -> [w580] mode=indexing
          tunnel: [w571] -> w554
          tunnel: [w563] -> w550 mode=indexing
          i -> [w573]
          w564 = 30 ("x")
          n238 = Index Array(array=w580, index #1=0 ("index"), index #2=1 ("index")) -> (element #1=w576:dbl, element #2=w575:dbl)
          n239 = To Long Integer(number=w576) -> (32bit integer=w568:i32)
          n240 = To Long Integer(number=w575) -> (32bit integer=w565:i32)
          n241 = Subtract(x=w565, y=w564) -> (x-y=w566:i32)
          n242 = Add(x=w564, y=w568) -> (x+y=w567:i32)
          n243 = Bundle By Name(cluster=cluster{"X-Coordinate":i32, "Y-Coordinate":i32} {"X-Coordinate"=0, "Y-Coordinate"=0}, "X-Coordinate"=w567, "Y-Coordinate"=w566) -> (w563:cluster{"X-Coordinate":i32, "Y-Coordinate":i32})
          n244 = Increment(x=w573) -> (x+1=w572:i32)
          n245 = Format Into String(w572) -> (resulting string=w582:string)  [unwired: 3 in, 1 out]
          n246 = call "IMAQ Overlay Text"("Text Color (black)"=u32 16711680, "error in (no error)"=w574, "String"=w582, "Origin"=w563, "Image"=w570) -> ("error out"=w571:errorcluster, "Image Out"=w569:T1)  [unwired: 5 in]
        }
        n247 = call "IMAQ Merge Overlay"("error in (no error)"=w554, "Image Src"=w553) -> ("error out"=w555:errorcluster, "Image Dst Out"=w552:T1)  [unwired: 8 in]
        "Droplet Lables" <- w552
        n248 = Bundle By Name(cluster=w559, "Camera Cluster.Lable Image"=w552, "Data Out Cluster.Lable coordinates"=w550) -> (w558:T2)
        n249 = call <vilib>:"Add State(s) to Queue__jki_lib_state_machine.vi"("State(s) in (\"\")"=w562) -> ("States Out"=w561:string)  [unwired: 14 in]
      }
      frame "---------- Arduino ----------" {
        # "Template Separator\n(You can make a copy of, or modify, this frame)"
        n250 = call <vilib>:"Add State(s) to Queue__jki_lib_state_machine.vi"("State(s) in (\"\")"=w586) -> ("States Out"=w585:string)  [unwired: 14 in]
      }
      frame "Arduino: Initialize" {
        # "Template Separator\n(You can make a copy of, or modify, this frame)"
        n251 = call "Arduino_Initialization_GCFS.vi"("error in"=w592) -> ("error out"=w591:errorcluster, "Connection"=w587:bool, "VISA Arduino"=w588:refnum<visa-resource-name>)  [unwired: 7 in]
        "UNO Connection" <- w587
        n252 = Bundle By Name(cluster=w590, "Arduino.Port"=w588, "Arduino.Connection"=w587) -> (w589:T2)
        n253 = call <vilib>:"Add State(s) to Queue__jki_lib_state_machine.vi"("State(s) in (\"\")"=w594) -> ("States Out"=w593:string)  [unwired: 14 in]
      }
      frame "Arduino: State" {
        # "Template Separator\n(You can make a copy of, or modify, this frame)"
        n254 = Unbundle By Name(w600) -> ("Arduino.Port"=w602:refnum<visa-resource-name>, "Arduino.Connection"=w601:bool, "Arduino.State"=w595:string)
        n255 = call "Arduino_control_GCFS.vi"("error in (no error)"=w597, "Arguments"=w595, "Connection"=w601, "Port"=w602) -> ("error out"=w596:errorcluster, "Connection"=w598:bool)
        n256 = Bundle By Name(cluster=w600, "Arduino.Connection"=w598) -> (w599:T2)
        n257 = call <vilib>:"Add State(s) to Queue__jki_lib_state_machine.vi"("State(s) in (\"\")"=w604) -> ("States Out"=w603:string)  [unwired: 14 in]
      }
      frame "Arduino: Terminate" {
        # "Template Separator\n(You can make a copy of, or modify, this frame)"
        n258 = Unbundle By Name(w608) -> ("Arduino.Port"=w609:refnum<visa-resource-name>, "Arduino.Connection"=w610:bool)
        n259 = case shown="True" w610 {
          tunnel: w609 -> [_ w616]
          tunnel: w608 -> [w614 w620]
          tunnel: [w614 w619] -> w605
          tunnel: [w613 w618] -> w606
          tunnel: w607 -> [w613 w617]
          frame False {
          }
          frame True {
            w615 = FALSE ("Connections.Arduino.Connected")
            n260 = VISA Close(VISA resource name=w616, error in (no error)=w617) -> (error out=w618:errorcluster)
            n261 = local write "UNO Connection"(w615) -> ()
            n262 = Bundle By Name(cluster=w620, "Arduino.Connection"=w615, "Active"=w615) -> (w619:T2)
          }
        }
        n263 = call <vilib>:"Add State(s) to Queue__jki_lib_state_machine.vi"("State(s) in (\"\")"=w612) -> ("States Out"=w611:string)  [unwired: 14 in]
      }
      frame "---------- PSU ----------" {
        # "Template Separator\n(You can make a copy of, or modify, this frame)"
        n264 = call <vilib>:"Add State(s) to Queue__jki_lib_state_machine.vi"("State(s) in (\"\")"=w624) -> ("States Out"=w623:string)  [unwired: 14 in]
      }
      frame "PSU: Initialize" {
        # "Template Separator\n(You can make a copy of, or modify, this frame)"
        n265 = call "Connect_PSU_GCFS.vi"("error in (no error)"=w628, 7:w630) -> ("error out"=w627:errorcluster, "State out"=w626:string, "Connected?"=→"PSU Connection":bool, "output cluster"=w629:T2)  [unwired: 2 in]
        n266 = call <vilib>:"Add State(s) to Queue__jki_lib_state_machine.vi"("State(s) in Front (\"\")"=w626, "State(s) in (\"\")"=w632) -> ("States Out"=w631:string)  [unwired: 13 in]
      }
      frame "PSU: Mode" {
        # "Template Separator\n(You can make a copy of, or modify, this frame)"
        n267 = Unbundle By Name(w643) -> ("PSU.Connection"=w645:bool, "PSU.Port"=w644:refnum<visa-resource-name>, "PSU.State"=w638:string)
        n268 = Equal?(x=w638, y="OFF") -> (x = y?=w636:bool)
        n269 = Select(t="1", s=w636, f="0") -> (s? t:f=w634:string)
        n270 = Concatenate Strings("SOUT", w634) -> (w639:string)
        n271 = call "PSUController_GCFS.vi"("error in (no error)"=w642, "VISA.PSU"=w644, "Output"=w639, "PSU.Connected"=w645) -> ("error out"=w641:errorcluster)  [unwired: 1 in, 1 out]
        n272 = call <vilib>:"Add State(s) to Queue__jki_lib_state_machine.vi"("State(s) in (\"\")"=w647) -> ("States Out"=w646:string)  [unwired: 14 in]
      }
      frame "PSU: Max Output" {
        # "Template Separator\n(You can make a copy of, or modify, this frame)"
        n273 = Unbundle By Name(w654) -> ("PSU.Connection"=w653:bool, "PSU.Port"=w652:refnum<visa-resource-name>)
        n274 = call "PSU_VOUT_Converter.vi"("Output %"=70.0) -> ("decimal integer string"=w649:string)  [unwired: 1 out]
        n275 = call "PSUController_GCFS.vi"("error in (no error)"=w651, "VISA.PSU"=w652, "Output"=w649, "PSU.Connected"=w653) -> ("error out"=w650:errorcluster)  [unwired: 1 in, 1 out]
        n276 = call <vilib>:"Add State(s) to Queue__jki_lib_state_machine.vi"("State(s) in (\"\")"=w656) -> ("States Out"=w655:string)  [unwired: 14 in]
      }
      frame "PSU: Min Output" {
        # "Template Separator\n(You can make a copy of, or modify, this frame)"
        n277 = Unbundle By Name(w663) -> ("PSU.Connection"=w662:bool, "PSU.Port"=w661:refnum<visa-resource-name>)
        n278 = call "PSU_VOUT_Converter.vi"("Output %"=0.0) -> ("decimal integer string"=w658:string)  [unwired: 1 out]
        n279 = call "PSUController_GCFS.vi"("error in (no error)"=w660, "VISA.PSU"=w661, "Output"=w658, "PSU.Connected"=w662) -> ("error out"=w659:errorcluster)  [unwired: 1 in, 1 out]
        n280 = call <vilib>:"Add State(s) to Queue__jki_lib_state_machine.vi"("State(s) in (\"\")"=w665) -> ("States Out"=w664:string)  [unwired: 14 in]
      }
      frame "PSU: Terminate" {
        # "Template Separator\n(You can make a copy of, or modify, this frame)"
        n281 = Unbundle By Name(w671) -> ("PSU.Port"=w668:refnum<visa-resource-name>, "PSU.Connection"=w670:bool)
        n282 = call "PSUController_GCFS.vi"("error in (no error)"=w667, "VISA.PSU"=w668, "Output"="SOUT1", "PSU.Connected"=w670) -> ("error out"=w669:errorcluster)  [unwired: 1 in, 1 out]
        n283 = case shown="True" w670 {
          tunnel: w668 -> [_ w680]
          tunnel: w671 -> [w676 w682]
          tunnel: [w676 w681] -> _
          tunnel: [w675 w679] -> w672
          tunnel: w669 -> [w675 w678]
          frame False {
          }
          frame True {
            w677 = FALSE ("Connections.cDAQ.Connected")
            n284 = VISA Close(VISA resource name=w680, error in (no error)=w678) -> (error out=w679:errorcluster)
            n285 = Bundle By Name(cluster=w682, "PSU.Connection"=w677) -> (w681:T2)
            n286 = local write "PSU Connection"(w677) -> ()
          }
        }
        n287 = call <vilib>:"Add State(s) to Queue__jki_lib_state_machine.vi"("State(s) in (\"\")"=w674) -> ("States Out"=w673:string)  [unwired: 14 in]
      }
      frame "---------- cDAQ ----------" {
        # "Template Separator\n(You can make a copy of, or modify, this frame)"
        n288 = call <vilib>:"Add State(s) to Queue__jki_lib_state_machine.vi"("State(s) in (\"\")"=w686) -> ("States Out"=w685:string)  [unwired: 14 in]
      }
      frame "cDAQ: Scan" {
        # "Template Separator\n(You can make a copy of, or modify, this frame)"
        n289 = for {
          N: 5 -> [_]
          tunnel: "cDAQ" -> [w699]
          tunnel: "Mod1/ai1" -> [w706]
          shift-right: [w703] -> w687
          shift-left: "N/A" -> [w702]
          i -> [w708]
          n290 = Increment(x=w708) -> (x+1=w707:i32)
          n291 = Number To Decimal String(number=w707) -> (decimal integer string=w698:string)  [unwired: 1 in]
          n292 = Concatenate Strings(w699, w698) -> (w697:string)
          n293 = Concatenate Strings(w699, w698, w706) -> (w705:string)
          n294 = call-poly <vilib>:"DAQmx Create Virtual Channel.vi"("task in"=refnum<k21> refnum, "physical channels"=w705) -> ("task out"=w701:refnum<k21>, "error out"=w704:errorcluster)  [unwired: 12 in]
          n295 = case shown="No Error" w704 {
            tunnel: w697 -> [w710 _]
            tunnel: [w710 w712] -> w703
            tunnel: w702 -> [_ w712]
            tunnel: w701 -> [w709 w711]
            frame No Error {
              n296 = call <vilib>:"DAQmx Clear Task.vi"("task in"=w709) -> ()  [unwired: 14 in, 1 out]
            }
            frame Error {
              n297 = call <vilib>:"DAQmx Clear Task.vi"("task in"=w711) -> ()  [unwired: 14 in, 1 out]
            }
          }
        }
        n298 = Bundle By Name(cluster=w689, "cDAQ.ID"=w687) -> (w688:T2)
        n299 = call <vilib>:"Add State(s) to Queue__jki_lib_state_machine.vi"("State(s) in (\"\")"=w696) -> ("States Out"=w695:string)  [unwired: 14 in]
      }
      frame "cDAQ: Initialize" {
        w724 = 10143 items=["Deg C"=10143, "Deg F"=10144, "Kelvins"=10325, "Deg R"=10145, "From Custom Scale"=10065] ("units")
        w725 = 4 items=["2-Wire"=2, "3-Wire"=3, "4-Wire"=4] ("resistance configuration")
        w728 = 10200 items=["Internal"=10200, "External"=10167, "None"=10230] ("current excitation source")
        w729 = 10071 items=["Pt3750"=12481, "Pt3851"=10071, "Pt3911"=12482, "Pt3916"=10069, "Pt3920"=10053, "Pt3928"=12483, "Custom"=10137] ("rtd type")
        # "Template Separator\n(You can make a copy of, or modify, this frame)"
        n300 = Unbundle By Name(w719) -> ("cDAQ.ID"=w732:string)
        n301 = Concatenate Strings(w732, "Mod1/ai1") -> (w720:string)
        n302 = call-poly <vilib>:"DAQmx Create Virtual Channel.vi"("task in"=refnum<k21> refnum, "maximum value"=80.0, "minimum value"=-50.0, "resistance configuration"=w725, "physical channels"=w720, "r0"=100.0, "name to assign"="temp1", "units"=w724, "current excitation value"=0.0005, "error in"=w717, "current excitation source"=w728, "rtd type"=w729) -> ("task out"=w715:refnum<k21>, "error out"=w716:errorcluster)  [unwired: 2 in]
        n303 = Unbundle By Name(w716) -> ("status"=w714:bool)
        n304 = Not(x=w714) -> (.not. x?=w713:bool)
        "cDAQ Connection" <- w713
        n305 = Bundle By Name(cluster=w719, "cDAQ.Task"=w715, "cDAQ.Connection"=w713) -> (w718:T2)
        n306 = call <vilib>:"Add State(s) to Queue__jki_lib_state_machine.vi"("State(s) in (\"\")"=w734) -> ("States Out"=w733:string)  [unwired: 14 in]
      }
      frame "cDAQ: Terminate" {
        # "Template Separator\n(You can make a copy of, or modify, this frame)"
        n307 = Unbundle By Name(w739) -> ("cDAQ.Task"=w737:refnum<k21>, "cDAQ.Connection"=w738:bool)
        n308 = case shown="True" w738 {
          tunnel: w737 -> [_ w750]
          tunnel: w739 -> [w744 w749]
          tunnel: [w744 w748] -> w740
          tunnel: [w743 w747] -> w735
          tunnel: w736 -> [w743 w746]
          frame False {
          }
          frame True {
            w745 = FALSE ("Connections.cDAQ.Connected")
            n309 = call <vilib>:"DAQmx Clear Task.vi"("task in"=w750, "error in"=w746) -> ("error out"=w747:errorcluster)  [unwired: 13 in]
            n310 = local write "cDAQ Connection"(w745) -> ()
            n311 = Bundle By Name(cluster=w749, "cDAQ.Connection"=w745) -> (w748:T2)
          }
        }
        n312 = call <vilib>:"Add State(s) to Queue__jki_lib_state_machine.vi"("State(s) in (\"\")"=w742) -> ("States Out"=w741:string)  [unwired: 14 in]
      }
    }
    n313 = call <extravilib>:"Write.vi"("element"=w5) -> ("channel"=w6:T11)  [unwired: 1 out]
  }
  n314 = while {
    tunnel: w1 -> [w760]
    i -> [w755]
    stop <- w756 stop-if-true
    n315 = call <extravilib>:"Read.vi"("channel"=w760) -> ("element"=w758:T2)  [unwired: 1 in, 1 out]
    n316 = feedback #1() -> (w751:bool)  [unwired: 1 in]
    n317 = Unbundle By Name(w758) -> ("Cool A."=w752:bool, "Active"=w753:bool, "Exit"=w757:bool)
    n318 = feedback-in #1(w752) -> ()
    n319 = call "Timing_GCFS.vi"(0:w758) -> ("Sample dt (ms)"=w759:i64, "Sample dt (s)"=w754:dbl)
    n320 = case shown="True" w753 {
      tunnel: w760 -> [_ w770]
      tunnel: w759 -> [_ w769]
      tunnel: w757 -> [w762 w768]
      tunnel: [w762 w767] -> w756
      tunnel: w754 -> [_ w766]
      tunnel: w752 -> [_ w765]
      tunnel: w751 -> [_ w763]
      frame False {
        n321 = Wait (ms)(milliseconds to wait=u32 100) -> ()  [unwired: 1 out]
      }
      frame True {
        # "Pixel analasys loop"
        n322 = case shown="True" w765 {
          selector: w765 -> [_ w808]
          tunnel: w770 -> [w798 w812]
          tunnel: w769 -> [w784 w810]
          tunnel: w768 -> [w799 w811]
          tunnel: [w799 w811] -> w767
          tunnel: w766 -> [w793 _]
          tunnel: [w783 w809] -> w764
          tunnel: w763 -> [w775 _]
          frame False {
            n323 = call <extravilib>:"Read.vi"("channel"=w798) -> ("element"=w797:T2)  [unwired: 1 in, 1 out]
            n324 = Wait (ms)(milliseconds to wait=w784) -> ()  [unwired: 1 out]
            n325 = Unbundle By Name(w797) -> ("PSU.Connection"=w786:bool, "PSU.Port"=w788:refnum<visa-resource-name>, "cDAQ.Connection"=w795:bool, "cDAQ.Task"=w796:refnum<k21>, "Data In Cluster.Control.HeatingPID gains"=w772:T8, "Arduino.Connection"=w785:bool, "Arduino.Port"=w787:refnum<visa-resource-name>)
            n326 = case shown="True" w795 {
              tunnel: w796 -> [_ w806]
              tunnel: [15.0 ("data") w805] -> w771
              tunnel: [errorcluster {"status"=TRUE, "code"=0, "source"="Temps reading error. Not active state"} ("error out") w804] -> w789
              frame False {
              }
              frame True {
                n327 = call-poly <vilib>:"DAQmx Read.vi"("task/channels in"=w806) -> ("data"=w805:dbl, "error out"=w804:errorcluster)  [unwired: 12 in, 1 out]
              }
            }
            "Waveform Chart" <- w771
            n328 = local write "Temperature"(w771) -> ()
            n329 = Less?(x=w771, y=10.0) -> (x < y?=w773:bool)
            n330 = case shown="True" w773 {
              tunnel: ["Repeat" "Heat"] -> w780
              frame False {
              }
              frame True {
              }
            }
            n331 = First Call?() -> (First Call?: T/F=w774:bool)
            n332 = Compound Arithmetic op=OR(w775, w774, w773) -> (w776:bool)
            n333 = Greater?(x=w771, y=25.0) -> (0:w779:bool)
            n334 = call-poly <vilib>:"PID.vi"("reinitialize? (F)"=w776, "output range"=cluster{"output high":dbl, "output low":dbl} {"output high"=100.0, "output low"=0.0}, "dt (s)"=w793, "PID gains"=w772, "process variable"=w771, "setpoint"=20.0) -> ("output"=w791:dbl)  [unwired: 4 in, 1 out]
            n335 = Select(t="Off", s=w779, f=w780) -> (s? t:f=w781:string)
            n336 = call "Arduino_control_GCFS.vi"("error in (no error)"=w789, "Arguments"=w781, "Connection"=w785, "Port"=w787) -> ("error out"=w790:errorcluster)  [unwired: 1 out]
            n337 = call "PSU_CMD_GCFS.vi"("error in"=w790, "Connection"=w786, "Port"=w788, "output"=w791) -> ("error out"=w783:errorcluster)  [unwired: 2 out]
          }
          frame True {
            w807 = string[][] []
            n338 = while {
              tunnel: w812 -> [w842]
              shift-right: [w829] -> w809
              shift-left: _ -> [w837]
              shift-right: [w816] -> _
              shift-left: w807 -> [w813]
              shift-right: [w815] -> _
              shift-left: w807 -> [w814]
              shift-right: [w820] -> _
              shift-left: _ -> [_]
              tunnel: w810 -> [w827]
              tunnel: w808 -> [w819]
              i -> [w821]
              stop <- w826 stop-if-true
              n339 = Wait (ms)(milliseconds to wait=w827) -> ()  [unwired: 1 out]
              n340 = call "Is Value Changed.vim"("value"=w819) -> ("changed or first call?"=w818:bool)
              n341 = call <extravilib>:"Read.vi"("channel"=w842) -> ("element"=w835:T2)  [unwired: 1 in, 1 out]
              n342 = Select(t="Cool", s=w818, f="Repeat" ("Arguments")) -> (s? t:f=w823:string)
              n343 = Unbundle By Name(w835) -> ("Data Out Cluster.Que"=w836:refnum<queue>, "Arduino.Port"=w839:refnum<visa-resource-name>, "Arduino.Connection"=w838:bool, "Exit"=w840:bool, "Active"=w828:bool)  [unwired: 1 out]
              n344 = call "Arduino_control_GCFS.vi"("error in (no error)"=w837, "Arguments"=w823, "Connection"=w838, "Port"=w839) -> ("error out"=w834:errorcluster, "Connection"=w825:bool)
              n345 = Not(x=w828) -> (.not. x?=w841:bool)
              n346 = local write "UNO Connection"(w825) -> ()
              n347 = Or(x=w840, y=w841) -> (x .or. y?=w826:bool)
              n348 = call "Sensors_GCFS.vi"(0:w835, "Value_Array_In"=w813, "Freezing_points"=w814, "reinitialize? (F)"=w818, "error in"=w834) -> ("Image Out"=w833:T1, "date/time string"=w832:string, "Temperature"=w820:dbl, "Freezing data"=w831:bool, "Value_Array_Out"=w815:string[][], "Freezing_points_Out"=w816:string[][], "valid?"=→"valid?":bool, "error out"=w830:errorcluster)  [unwired: 3 in]
              "Frezz Image" <- w833
              "Temperature" <- w820
              n349 = call "Que_elements_GCFS.vi"("Pixel values"=w816, "queue"=w836, "Freezing points"=w815, "error in (no error)"=w830, "Snap timestamp"=w832, "Image To Save"=w833, "FreezingData"=w831) -> ("error out"=w829:errorcluster)  [unwired: 2 in, 2 out]
              "Data run" <- w821
            }
          }
        }
        "error out" <- w764
      }
    }
    "Data Loop" <- w755
  }
  n350 = while {
    tunnel: w1 -> [w850]
    i -> [w848]
    stop <- w844 stop-if-true
    # "Append to file loop"
    n351 = call <extravilib>:"Read.vi"("channel"=w850) -> ("element"=w849:T2)  [unwired: 1 in, 1 out]
    n352 = Unbundle By Name(w849) -> ("Data Out Cluster.Que"=w847:refnum<queue>, "Data In Cluster.Images.Sample folder path"=w846:path, "Active"=w843:bool, "Exit"=w845:bool)
    n353 = case shown="True" w843 {
      tunnel: w847 -> [_ w860]
      tunnel: w846 -> [_ w857]
      tunnel: w845 -> [w851 w855]
      tunnel: [w851 w854] -> w844
      frame False {
        n354 = Wait (ms)(milliseconds to wait=u32 100) -> ()  [unwired: 1 out]
      }
      frame True {
        n355 = Dequeue Element(queue=w860, timeout in ms (-1)=50) -> (element=w858:T6, timed out?=w856:bool)  [unwired: 1 in, 2 out]
        n356 = Not(x=w856) -> (.not. x?=w853:bool)
        n357 = case shown="True" w853 {
          tunnel: w857 -> [_ w875]
          tunnel: w858 -> [_ w869]
          tunnel: w855 -> [w861 w863]
          tunnel: [w861 w863] -> w854
          frame False {
            n358 = Wait (ms)(milliseconds to wait=u32 50) -> ()  [unwired: 1 out]
          }
          frame True {
            n359 = Unbundle By Name(w869) -> ("Freezing points"=w868:string[][], "Pixel values"=w867:string[][], "FreezingData"=w866:bool, "Image To Save"=w864:T1, "Snap timestamp"=w865:string)  [unwired: 1 out]
            n360 = Search and Replace String(replace all?=TRUE ("replace all? (F)"), input string=w865, search string=":", replace string=";" ("replace string (\"\")")) -> (result string=w873:string)  [unwired: 4 in, 3 out]
            n361 = Path To String(path=w875) -> (string=w880:string)
            n362 = Concatenate Strings(w880, "\\" ("string")) -> (w879:string)
            n363 = Concatenate Strings(w879, "Sample_Image_" ("string"), w873, ".PNG" ("string")) -> (w884:string)
            n364 = String To Path(string=w884) -> (path=w882:path)
            n365 = call-poly "IMAQ Write File 2"("File Path"=w882, "Image"=w864) -> ("error out"=w877:errorcluster)  [unwired: 8 in, 1 out]
            n366 = call "Save_Files_GCFS.vi"("error in"=w877, "Enum"=enum16{"Freezing_Data", "Sample_Data"}."Sample_Data", "Array"=w867, "file path (use dialog)"=w875) -> ("error out"=w876:errorcluster)  [unwired: 1 in, 1 out]
            n367 = case shown="True" w866 {
              tunnel: w876 -> [w885 w888]
              tunnel: w868 -> [_ w891]
              tunnel: w875 -> [_ w890]
              tunnel: [w885 w889] -> _
              frame False {
              }
              frame True {
                n368 = call "Stall Data Flow.vim"("value in"=w888, "milliseconds to wait"=u32 10) -> ("value out"=w887:errorcluster)  [unwired: 1 out]
                n369 = call "Save_Files_GCFS.vi"("error in"=w887, "Enum"=enum16{"Freezing_Data", "Sample_Data"}."Freezing_Data", "Array"=w891, "file path (use dialog)"=w890) -> ("error out"=w889:errorcluster)  [unwired: 1 in, 1 out]
              }
            }
          }
        }
      }
    }
    "Save loop" <- w848
  }
